vi "Striptest.vi"(1 "Simulation?":bool) -> ()   [LabVIEW 2013]
uses:
  InstrControl/Switching/Switching.lvclass
  InstrControl/SupplyControl/SupplyControl.lvclass
  InstrControl/ProbeStationControl/ProbeStationControl.lvclass
  InstrControl/LCRControl/LCRControl.lvclass
  general_VIs/globals/QC_MeasurementSetup.vi
  striptest/ProbePlan/ProbePlanParams.vi
  general_VIs/globals/QC_RunInformation.vi
  InstrControl/InstrumentSetup.vi
  <vilib>/regexp/Match Regular Expression.xnode
  InstrControl/InstrControl.lvclass
  InstrControl/ArduinoControl/ArduinoControl.lvclass
  <vilib>/Analysis/NI_AALBase.lvlib
panel:
  out "Tab Control":enum32{"Striptest Setup", "Striptest"}(tab)
  in  "Bias Voltage [V]":dbl=-150.0 format="%.1f"
  in  "Frequency [Hz] Setup":i32=1000 caption="Frequency [Hz]" format="%#.3p"
  in  "Minimum fraction\nof good strips":dbl=98.0 format="%.1g"
  in  "Quit":bool
  in  "Continue":bool
  in  "Measurement Configurations":bool
  in  "Pinholes Y/N":bool=TRUE
  in  "Capacitance Y/N":bool=TRUE
  in  "Resistance Y/N":bool=TRUE
  in  "Striptest SMU":string(combo)="Keithley 2410"
  in  "LCR Meter":string(combo)="WayneKerr 6440B"
  in  "Temperature":enum16{"Read Arduino", "Enter manually"}(ring)
  in  "Bias Supply":string(combo)="Keithley 2410"
  in  "Hardware Configurations":bool
  in  "DB Serial No. IN:":string caption="DB Serial No.:"
  in  "User:":string(combo)="Christoph"
  in  "Batch No. IN:":string caption="Batch No.:"
  in  "Device Category IN:":string(combo)="Short Strip" caption="Device Category:"
  in  "Wafer No. IN:":string caption="Wafer No.:"
  in  "From4":u16(ring)
  in  "From3":u16(ring)
  in  "From2":u16(ring)
  in  "From 1":u16(ring) caption="From"
  in  "To4":u16(ring)
  in  "To3":u16(ring)
  in  "To2":u16(ring)
  in  "To 1":u16(ring) caption="To"
  out "Region 1":string caption="Region"
  out "Region2":string
  out "Region3":string
  out "Region4":string
  in  "Enable1":bool
  in  "Enable4":bool
  in  "Enable2":bool
  in  "Enable3":bool
  in  "Pinhole Parameters IN":T1={"Base Voltage"=10.0, "Base Ramp [V/step]"=10.0, "Base Step [ms]"=1000, "High Voltage"=100.0, "High Ramp [V/step]"=100.0, "High Step [ms]"=1000} caption="Pinhole Measurement Parameters"
  in  "Manufacturer:":string(combo)="Hamamatsu"
  in  "Auto ReCheck":bool
  in  "Thresholds:":T2={"Current [nA]"=200.0, "Ccoupl Lo [pF/cm]"=20.0, "Ccoupl Hi [pF/cm]"=33.0, "Rbias Lo [MW]"=1.0, "Rbias Hi [MW]"=2.0}
  in  "Rolling\nCurrent Readout":bool=TRUE
  in  "settling\ndelay [ms]":i32=50
  in  "Pinhole Parameters":T1={"Base Voltage"=10.0, "Base Ramp [V/step]"=10.0, "Base Step [ms]"=1000, "High Voltage"=100.0, "High Ramp [V/step]"=100.0, "High Step [ms]"=1000}
  out "Bias On/Off:":bool
  in  "Auto quit &\nswitch off bias":bool
  out "Sensor No.:":string
  out "Device Category:":string
  out "DB Serial No.:":string
  out "Initiated:":string
  in  "ReCheck":bool
  in  "Save Data":bool
  in  "Abort":bool
  in  "Quit w/o saving":bool
  out "Probing Region:":string
  out "Probe Point:":string
  out "Current [nA]:":dbl
  out "Capacitance [pF]:":dbl
  out "Reistance [MW]:":dbl
  out "Last Probe at:":string
  out "Run Duration:":string
  out "Estimated Completion:":string
  out "Status:":string
  out "Probe Card Channels":i32=32
  in  "Show:":u16(ring)
  out "Defects":i32[][](graph)
  out "% OK:":dbl
  out "# total defects:":i32
  out "# probed":i32
  out "Bad Strip List":i32[](array[numeric])
  out "defect type array":i32[](array[numeric])
  out "Resistance [MW]":cluster{u32, i32, "Array OUT":dbl[]}(graph)
  out "Capacitance [pF]":cluster{u32, i32, "Array OUT":dbl[]}(graph)
  out "Current [nA]":cluster{u32, i32, "Array OUT":dbl[]}(graph)
  out "Current Reference 100V":dbl[](array[numeric])
  out "Current Reference 10V":dbl[](array[numeric])
  out "Single Needle":bool
  out "Z profile":i32[][](array[numeric])
  out "Start Temperature [°C]":dbl
  out "Last Temperature [°C]":dbl
  out "disabled channels":i32[](array[numeric])
  out "Module failed/passed":bool
  out "min scale array":i32[](array[numeric])
  out "max scale array":i32[](array[numeric])
  out "total strip number":u32
  out "Region Indices":i32[](array[numeric])
  out "Current Bias Voltage [V]":dbl
  out "Temperature Progression":T3
  out "probe points per region":i32[](array[numeric])
  # "University of \nCambridge"
  # "Sensor QC: Striptest"
  # "Current [nA]"
  # "Statistical information:"
  # "Pinholes:"
  # "Capacitance [pF]"
  # "Punchthroughs:"
  # "Shorts:"
  # "Opens:"
  # "Rpoly:"
  # "Resistance [MW]"
  # "Implant:"
  # "Current segment:"
  # "Ok  Pinhole at base  Pinhole after ramp  Short  Open  Rbias"
  # "Probe Range"
  # "Measurement Configuration"
  # "Hardware"
  # "DUT Description"
  # "Tests Included"
  # "Current status:"
  # "Measurement parameters:"
  # "DUT & Test Description:"
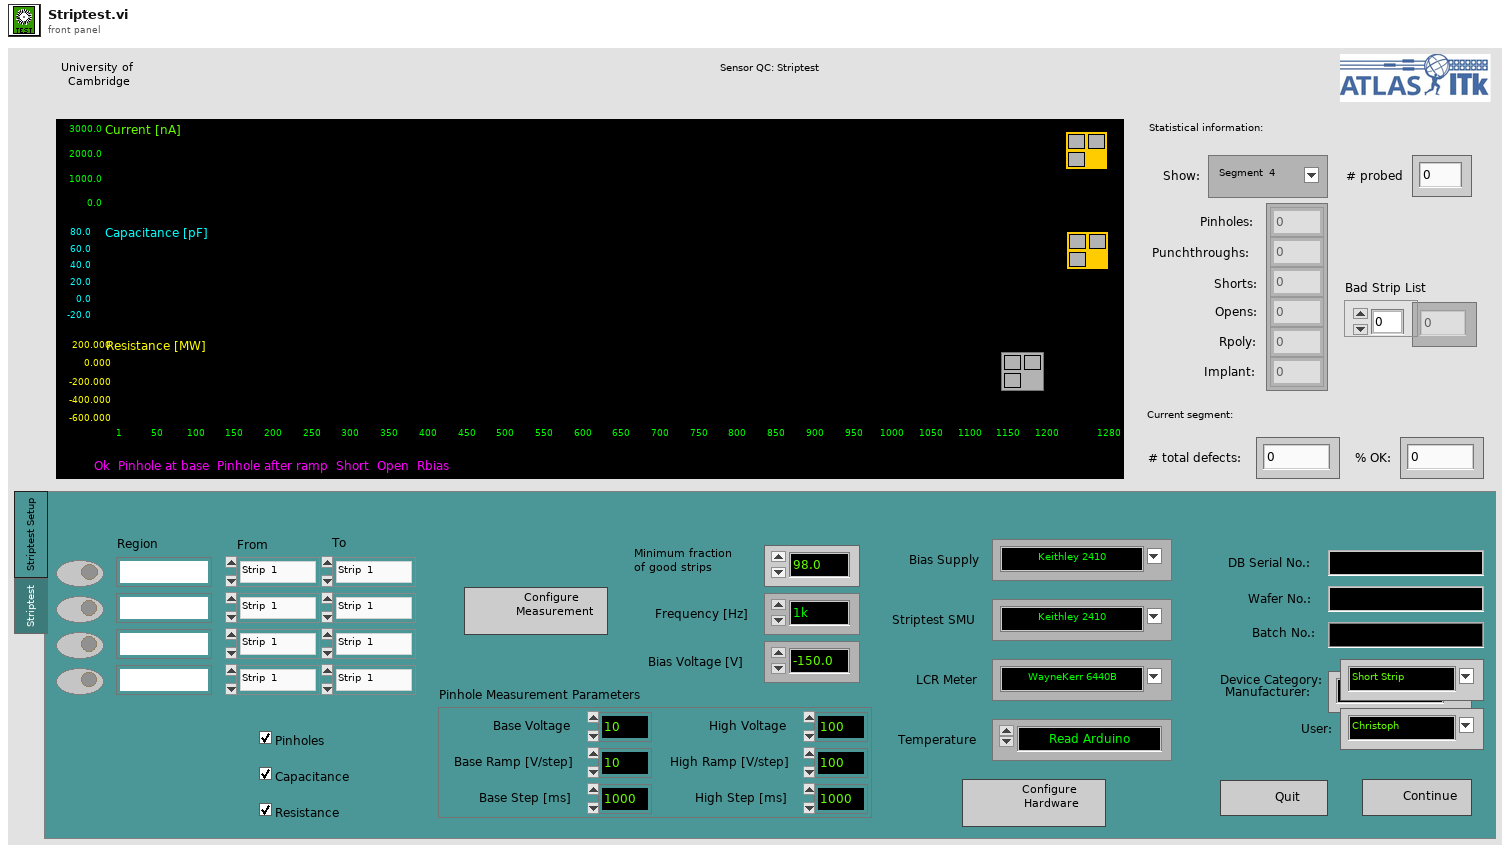
[diagram p1: front panel]
types:
  T1 = cluster{"Base Voltage":dbl, "Base Ramp [V/step]":dbl, "Base Step [ms]":i32, "High Voltage":dbl, "High Ramp [V/step]":dbl, "High Step [ms]":i32}
  T2 = cluster{"Current [nA]":dbl, "Ccoupl Lo [pF/cm]":dbl, "Ccoupl Hi [pF/cm]":dbl, "Rbias Lo [MW]":dbl, "Rbias Hi [MW]":dbl}
  T3 = cluster{"Time Array":string[], "Temperature Array [°C]":dbl[], "Humidity Array [RH %]":dbl[]}
  T4 = enum16{"Supply", "LCR", "Multimeter", "Switching"}
  T5 = enum16{"Reset", "Read Array", "Read Element", "Write Element", "Write Array", "Add Element", "Add Array"}
  T6 = enum16{"Reset", "Ground", "Striptest SMU", "Striptest LCR", "IV", "CV", "Interstrip Cap", "Interstrip Res"}
  T7 = enum16{"Reference measurement", "Baseline correcetion 10V", "Baseline correcetion 100V", "Nothing"}
  T8 = cluster{"Bias Supply":refnum<class "SupplyControl.lvclass">, "SMU":refnum<class "SupplyControl.lvclass">, "LCR":refnum<class "LCRControl.lvclass">, "ProbeStation":refnum<class "ProbeStationControl.lvclass">, "Arduino":refnum<class "ArduinoControl.lvclass">, "Measurement switch":refnum<class "Switching.lvclass">, "Probe Card Channels":i32, "Bias Voltage [V]":dbl, "First strip":i32, "Last strip":i32, "Base Voltage [V]":dbl, "Base Ramp Step [V]":dbl, "Base Ramp Interval [ms]":u32, "High Voltage [V]":dbl, "High Ramp Step [V]":dbl, "High Ramp Interval [ms]":u32, "AC frequency [Hz]":i32, "AC amplitude [V]":dbl, "RC Configuration":u16, "Single Needle":bool, "Temperature Readout":enum16{"Read Arduino", "Enter manually"}, "Fraction of good strips [%]":dbl, "Measurement switch used?":bool, "Matrix X Channels":cluster{"Mux1 C1":i32, "Mux1 C2":i32, "Mux2 C1":i32, "Mux2 C2":i32}, "Pinholes Y/N":bool, "Capacitance Y/N":bool, "Resistance Y/N":bool, "Bias Supply Name":string, "SMU Name":string, "LCR Name":string}
  T9 = cluster{"Institute":string, "Manufacturers":string[], "Devices":string[], "Serialnumbers Lookup DB":string, "Data directory":string, "Backup & screenshot directory":string, "List of known users":string[], "Measurement switch not used":bool, "Measurement Switch":string, "DUT Switch":string, "Rseries IV [MOhm]":string, "Rshunt IV [MOhm]":string, "Rseries CV [MOhm]":string, "DC blocking Cap [µF]":string, "Rseries LCR [MOhm]":string, "Rseries stability [MOhm]":string, "Rshunt stability [MOhm]":string, "Rseries striptest bias [MOhm]":string, "Rseries strip pinhole [MOhm]":string}
  T10 = cluster{"Sensor Serial No.:":string, "Wafer:":string, "Batch:":string, "Manufacturer:":string, "Device Category:":string, "Database Serial No.:":string, "Date Initiated:":string, "Time Initiated:":string, "Test":string, "Probeplan used:":string, "End of Run comment:":string, "User:":string, "Vbias SMU":string, "LCR":string, "Test SMU":string, "Test DMM":string}
  T11 = cluster{"Strip Number OUT":i32, "X0":i32, "Y0":i32, "X1":i32, "Y1":i32, "Xref":dbl, "Yref":dbl, "ProbePlan type":u32, "Inner pads offset":ext, "Outer pads offset":ext, "l_inner":ext, "l_outer":ext, "strip numbering":u16, "Device Orientation":ext, "Stagger offset":i32, "Yoffset":dbl, "Strip pitch":dbl, "Fiducail separation":dbl, "Radius":ext, "Relative strip angles":dbl, "Probeplan description":string, "ProbePlan array":cluster{"Region":string, "ProbePoints":cluster{"X":dbl, "Y":dbl, "Label":string, "CardViable?":bool}[]}[], "Test ProbePoints":cluster{"Regions Enabled":bool[], "From index":u32[], "To index":u32[]}}
  T12 = cluster{"Region":string, "ProbePoints":cluster{"X":dbl, "Y":dbl, "Label":string, "CardViable?":bool}[]}[]
  T13 = cluster{"VISA address":refnum<visa-resource-name>, "T sensor":enum16{"SHT", "DS"}, "Arduino":refnum<class "ArduinoControl.lvclass">}
  T14 = cluster{"X":dbl, "Y":dbl, "Label":string, "CardViable?":bool}[]
  T15 = cluster{"X":dbl, "Y":dbl, "Label":string, "CardViable?":bool}
  T16 = cluster{"pass Rate in %":dbl, "Bad channel list":i32[], "No of bad strips":i32, "Defect description list":i32[], "Number of defects per category":i32[], "Defect lists":string[], "No of channels":i32, "Defect Flag array OUT":i32[][]}
  T17 = cluster{"Hi Cap":dbl, "Lo Cap":dbl, "Current threshold":dbl, "Lo R":dbl, "Hi R":dbl}
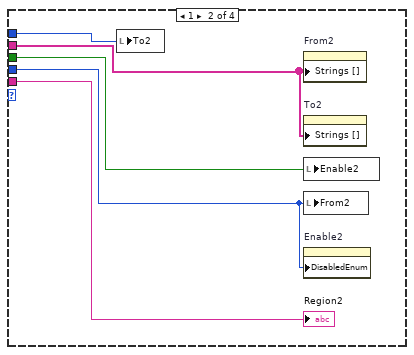
[diagram p3: hidden frame]
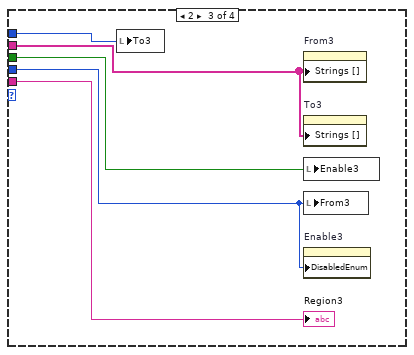
[diagram p4: hidden frame]
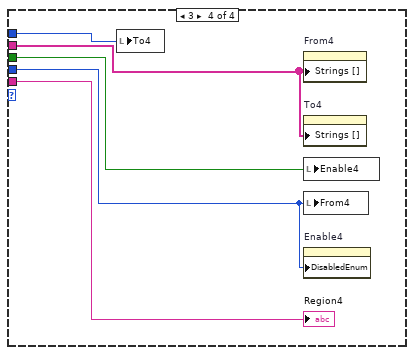
[diagram p5: hidden frame]
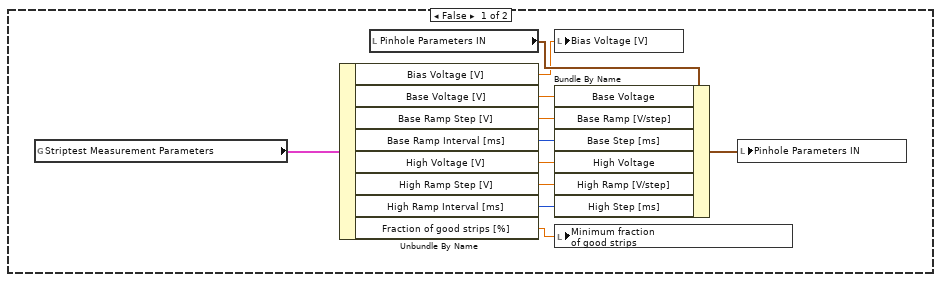
[diagram p7: hidden frame]
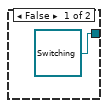
[diagram p9: hidden frame]
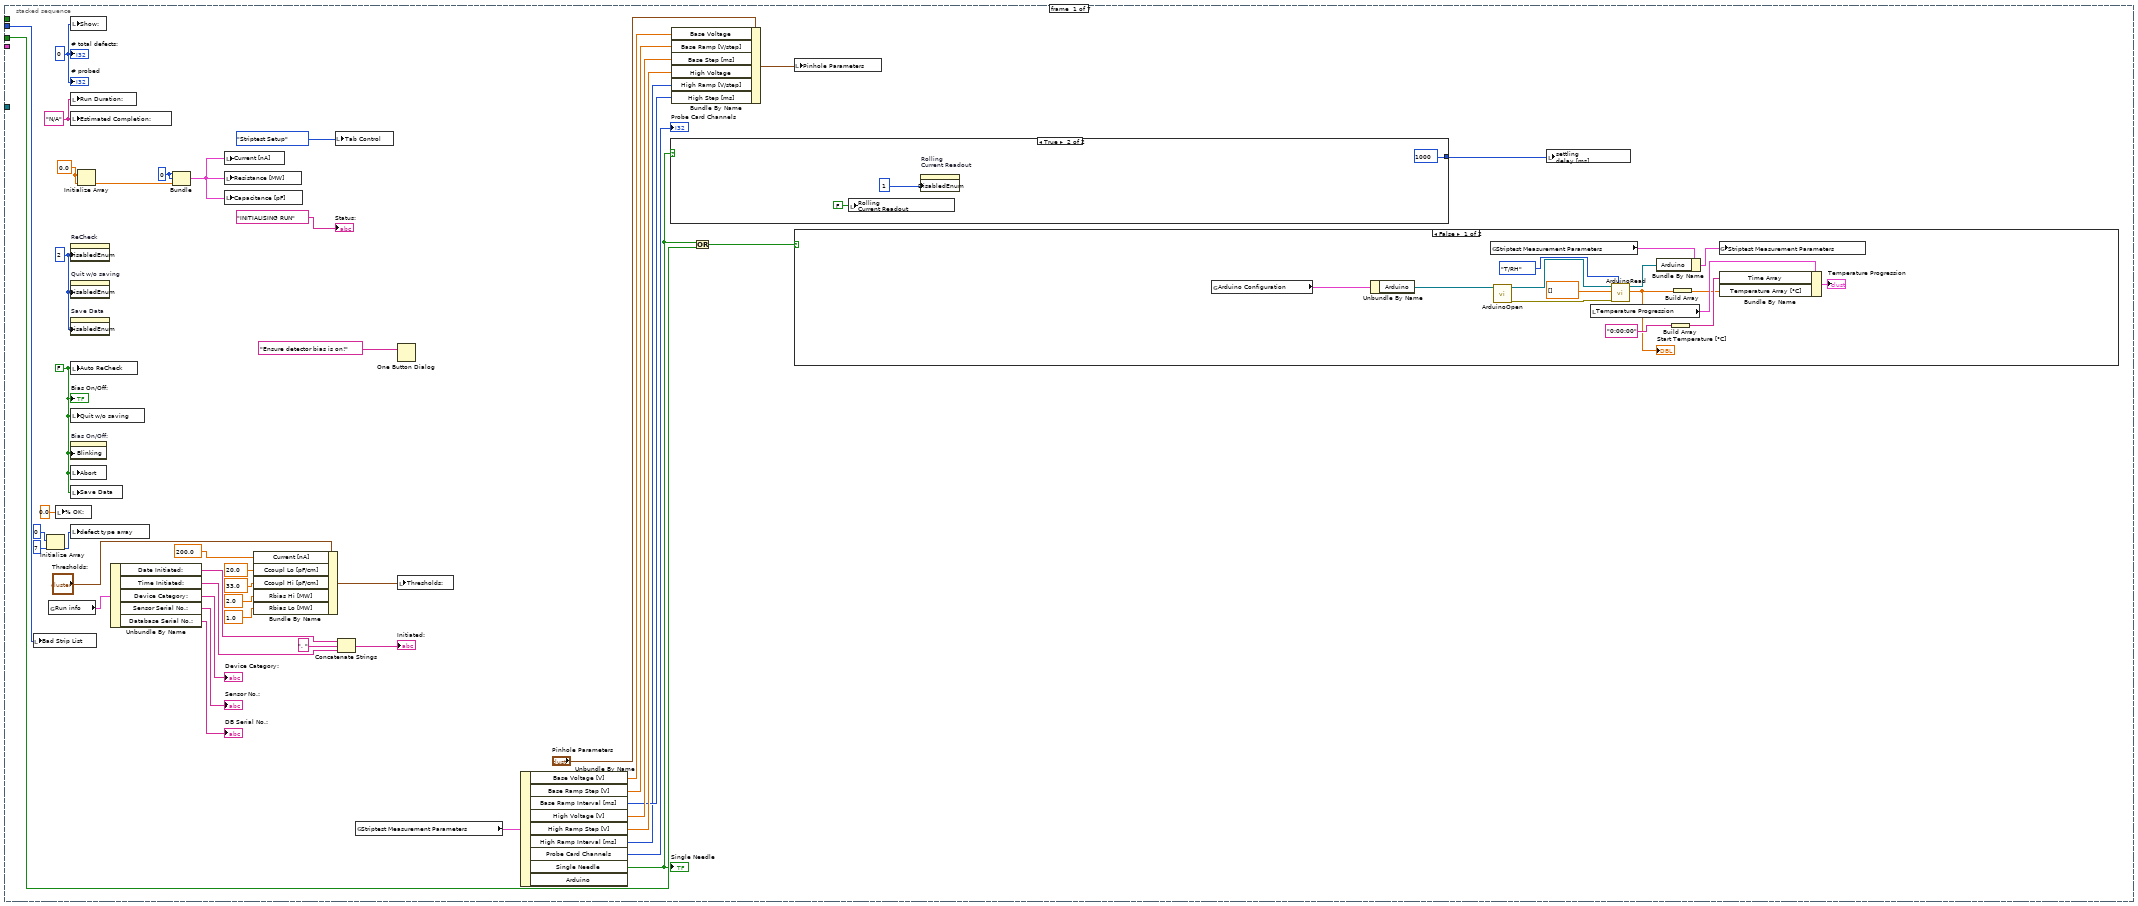
[diagram p10: hidden frame]
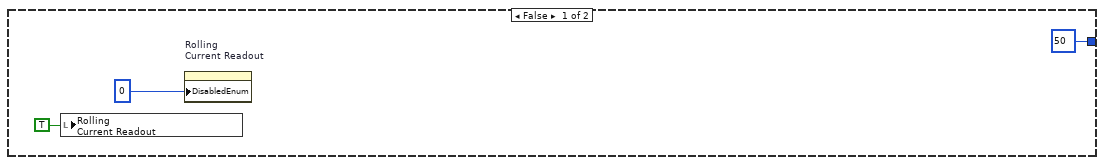
[diagram p11: hidden frame]
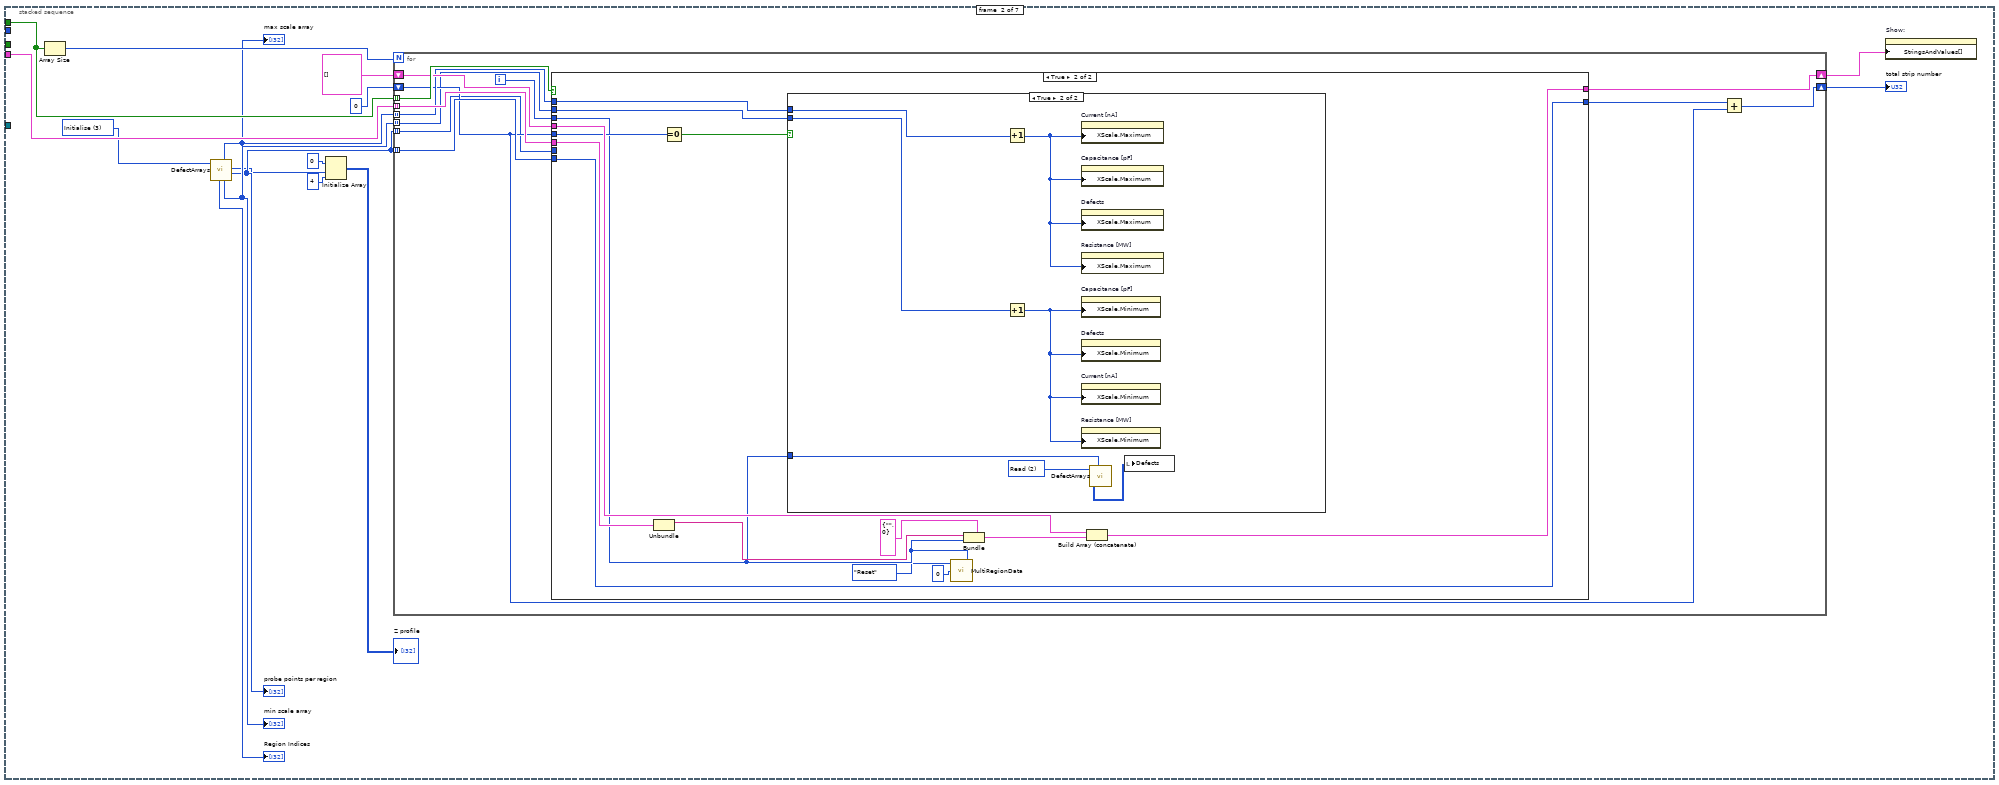
[diagram p13: hidden frame]
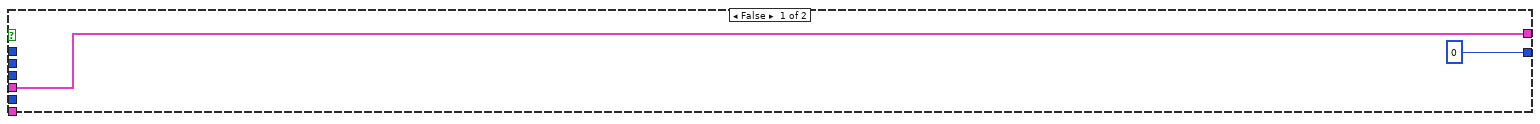
[diagram p14: hidden frame]
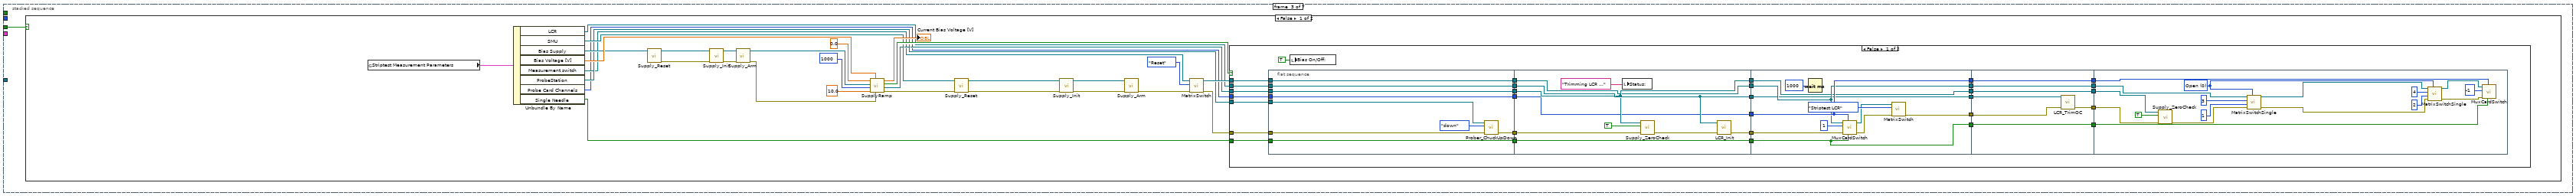
[diagram p16: hidden frame]
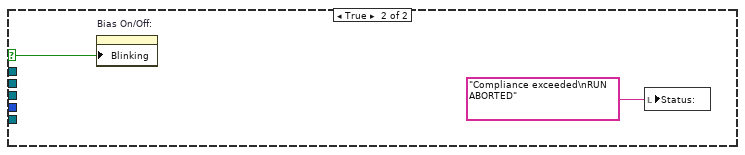
[diagram p17: hidden frame]
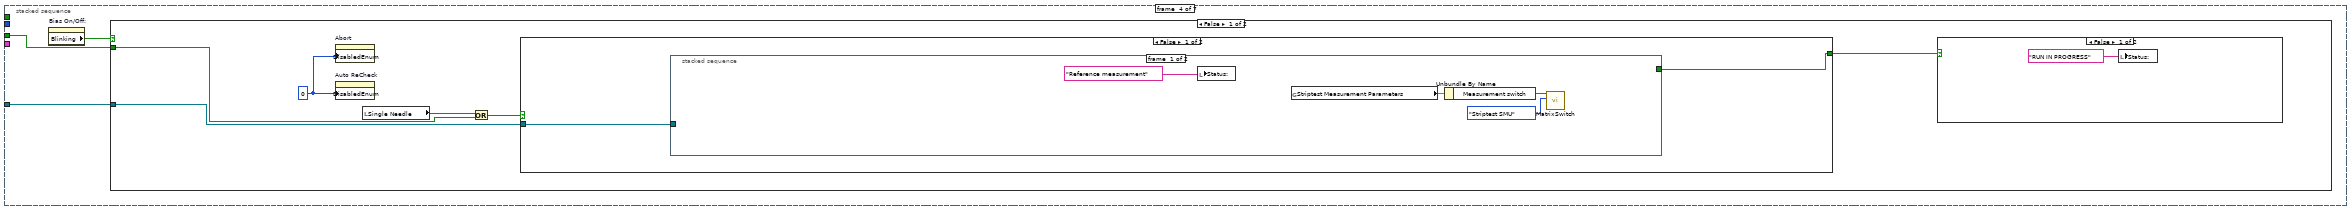
[diagram p19: hidden frame]
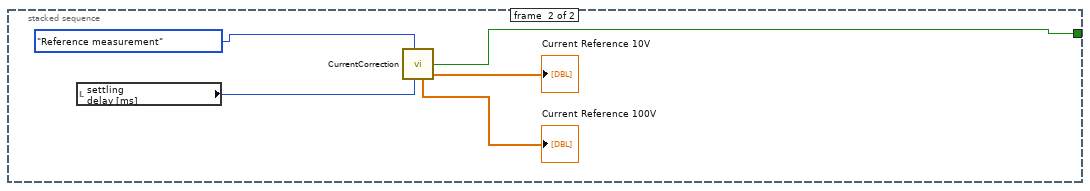
[diagram p20: hidden frame]
diagram:
  n1 = stacked-sequence {
    frame #0 {
      # "Striptest setup"
      n2 = flat-sequence {
        frame #0 {
          w5 = ""
          w6 = 2
          w7 = FALSE
          n3 = property on="Enable4" class="Bool (strict)"("DisabledEnum"=w6) -> ()  [unwired: 2 in, 2 out]
          n4 = property on="Enable1" class="Bool (strict)"("DisabledEnum"=w6) -> ()  [unwired: 2 in, 2 out]
          n5 = property on="Enable2" class="Bool (strict)"("DisabledEnum"=w6) -> ()  [unwired: 2 in, 2 out]
          n6 = property on="Enable3" class="Bool (strict)"("DisabledEnum"=w6) -> ()  [unwired: 2 in, 2 out]
          n7 = local write "Region 1"(w5) -> ()
          n8 = local write "Region2"(w5) -> ()
          n9 = local write "Region3"(w5) -> ()
          n10 = local write "Region4"(w5) -> ()
          n11 = local write "Enable2"(w7) -> ()
          n12 = local write "Enable1"(w7) -> ()
          n13 = local write "Enable3"(w7) -> ()
          n14 = local write "Enable4"(w7) -> ()
          n15 = call <vilib>:"Open Sessions.vi"() -> ("Array of Refnums"=w2:refnum<visa-resource-name>[])  [unwired: 2 in]
          n16 = for {
            tunnel: w2 -> [w13] mode=indexing
            tunnel: [w12] -> w1
            n17 = VISA Close(VISA resource name=w13) -> (error out=w12:errorcluster)  [unwired: 1 in]
          }
          n18 = call "SelectStriptestProber.vi"("error in (no error)"=w1) -> ("error out"=w8:errorcluster, "ProbeStationControl out"=w9:refnum<class "ProbeStationControl.lvclass">)  [unwired: 9 in]
          n19 = global read "QC_MeasurementSetup.vi" "Striptest Measurement Parameters"() -> (w11:T8)
          n20 = call "InitialiseProbeplan.vi"("error in (no error)"=w8, "ProbeStationControl in"=w9) -> ()  [unwired: 8 in, 2 out]
          n21 = Bundle By Name(cluster=w11, "ProbeStation"=w9) -> (w10:T8)
          n22 = global write "QC_MeasurementSetup.vi" "Striptest Measurement Parameters"(w10) -> ()
          n23 = call "GetLocalConfiguration.vi"() -> ()  [unwired: 3 in, 1 out]
          n24 = call "GetGlobalDefaultConfiguration.vi"("Read defaults?"=TRUE) -> ()  [unwired: 3 in]
          "Tab Control" <- enum32{"Striptest Setup", "Striptest"}."Striptest Setup" ("Tab Control")
        }
        frame #1 {
          n25 = flat-sequence {
            frame #0 {
              n26 = call "SerialNo.vi"("DB serial number IN"="", "Run uninterrupted?"=FALSE) -> ()  [unwired: 6 in, 2 out]
              n27 = global read "QC_RunInformation.vi" "LocalConfiguration"() -> (w49:T9)
              n28 = Unbundle By Name(w49) -> ("List of known users"=w51:string[], "Devices"=w46:string[], "Manufacturers"=w45:string[])
              n29 = property on="Device Category IN:" class="CmbBox"("Strings[]"=w46) -> ()  [unwired: 2 in, 2 out]
              n30 = property on="Manufacturer:" class="CmbBox"("Strings[]"=w45) -> ()  [unwired: 2 in, 2 out]
              n31 = Index Array(array=w46, index=0) -> (element=w43:string)
              n32 = Index Array(array=w45, index=0) -> (element=w44:string)
              n33 = property on="User:" class="CmbBox"("Strings[]"=w51, "AllowUndefStrs"=TRUE) -> ()  [unwired: 2 in, 2 out]
              n34 = local write "Device Category IN:"(w43) -> ()
              n35 = local write "Manufacturer:"(w44) -> ()
            }
            frame #1 {
              n36 = global read "QC_RunInformation.vi" "Run info"() -> (w54:T10)
              n37 = Unbundle By Name(w54) -> ("Wafer:"=w55:string, "Batch:"=w56:string, "Manufacturer:"=w57:string, "Device Category:"=w58:string, "Database Serial No.:"=w59:string)
              n38 = local write "Manufacturer:"(w57) -> ()
              n39 = local write "Device Category IN:"(w58) -> ()
              n40 = local write "DB Serial No. IN:"(w59) -> ()
              n41 = local write "Wafer No. IN:"(w55) -> ()
              n42 = local write "Batch No. IN:"(w56) -> ()
            }
          }
          n43 = global read "QC_RunInformation.vi" "Run info"() -> (w33:T10)
          n44 = call "InstrumentNames.vi"("Instrument type"=T4."Supply") -> ("error out"=w36:errorcluster, "Instrument names"=w38:string[])  [unwired: 9 in]
          n45 = global read "ProbePlanParams.vi" "ProbePlan Parameters IN"() -> (w42:T11)
          n46 = property on="Bias Supply" class="CmbBox"("Strings[]"=w38) -> ()  [unwired: 2 in, 2 out]
          n47 = property on="Striptest SMU" class="CmbBox"("Strings[]"=w38) -> ()  [unwired: 2 in, 2 out]
          n48 = Bundle By Name(cluster=w33, "Test"="STRIPTEST") -> (w34:T10)
          n49 = global write "QC_RunInformation.vi" "Run info"(w34) -> ()
          n50 = call "InstrumentNames.vi"("error in (no error)"=w36, "Instrument type"=T4."LCR") -> ("Instrument names"=w35:string[])  [unwired: 8 in, 1 out]
          n51 = property on="LCR Meter" class="CmbBox"("Strings[]"=w35) -> ()  [unwired: 2 in, 2 out]
          n52 = global read "QC_MeasurementSetup.vi" "Striptest Measurement Parameters"() -> (w32:T8)
          n53 = Unbundle By Name(w42) -> ("ProbePlan array"=w41:T12)
          n54 = Array Size(array=w41) -> (size(s)=w40:i32)
          n55 = for {
            N: w40 -> [_]
            tunnel: w41 -> [w61]
            tunnel: w41 -> [w65] mode=indexing
            i -> [w68]
            n56 = Unbundle(w65) -> ("Region"=w64:string)  [unwired: 1 out]
            n57 = call "GetLabels.vi"("Array"=w61) -> ("Strip Labels"=w60:string[])  [unwired: 3 out]
            n58 = Array Size(array=w60) -> (size(s)=w63:i32)
            n59 = Decrement(x=w63) -> (x-1=w62:i32)
            n60 = case shown="0, Default" w68 {
              tunnel: TRUE -> [w73 w77 w83 w88]
              tunnel: 0 -> [w69 w75 w79 w85]
              tunnel: w64 -> [w71 w76 w81 w86]
              tunnel: w60 -> [w70 w74 w80 w84]
              tunnel: w62 -> [w72 w78 w82 w87]
              frame 0, Default {
                n61 = local write "To 1"(w72) -> ()
                n62 = property on="To 1" class="Ring (strict)"("Strings []"=w70) -> ()  [unwired: 2 in, 2 out]
                n63 = property on="From 1" class="Ring (strict)"("Strings []"=w70) -> ()  [unwired: 2 in, 2 out]
                n64 = local write "Enable1"(w73) -> ()
                n65 = local write "From 1"(w69) -> ()
                n66 = property on="Enable1" class="Bool (strict)"("DisabledEnum"=w69) -> ()  [unwired: 2 in, 2 out]
                "Region 1" <- w71
              }
              frame 1 {
                n67 = local write "To2"(w78) -> ()
                n68 = property on="From2" class="Ring (strict)"("Strings []"=w74) -> ()  [unwired: 2 in, 2 out]
                n69 = property on="To2" class="Ring (strict)"("Strings []"=w74) -> ()  [unwired: 2 in, 2 out]
                n70 = local write "Enable2"(w77) -> ()
                n71 = local write "From2"(w75) -> ()
                n72 = property on="Enable2" class="Bool (strict)"("DisabledEnum"=w75) -> ()  [unwired: 2 in, 2 out]
                "Region2" <- w76
              }
              frame 2 {
                n73 = local write "To3"(w82) -> ()
                n74 = property on="From3" class="Ring (strict)"("Strings []"=w80) -> ()  [unwired: 2 in, 2 out]
                n75 = property on="To3" class="Ring (strict)"("Strings []"=w80) -> ()  [unwired: 2 in, 2 out]
                n76 = local write "Enable3"(w83) -> ()
                n77 = local write "From3"(w79) -> ()
                n78 = property on="Enable3" class="Bool (strict)"("DisabledEnum"=w79) -> ()  [unwired: 2 in, 2 out]
                "Region3" <- w81
              }
              frame 3 {
                n79 = local write "To4"(w87) -> ()
                n80 = property on="From4" class="Ring (strict)"("Strings []"=w84) -> ()  [unwired: 2 in, 2 out]
                n81 = property on="To4" class="Ring (strict)"("Strings []"=w84) -> ()  [unwired: 2 in, 2 out]
                n82 = local write "Enable4"(w88) -> ()
                n83 = local write "From4"(w85) -> ()
                n84 = property on="Enable4" class="Bool (strict)"("DisabledEnum"=w85) -> ()  [unwired: 2 in, 2 out]
                "Region4" <- w86
              }
            }
          }
          n85 = Unbundle By Name(w32) -> ("Probe Card Channels"=w31:i32, "Bias Voltage [V]"=w22:dbl, "Base Voltage [V]"=w28:dbl, "Base Ramp Step [V]"=w27:dbl, "Base Ramp Interval [ms]"=w26:u32, "High Voltage [V]"=w25:dbl, "High Ramp Step [V]"=w24:dbl, "High Ramp Interval [ms]"=w23:u32, "Single Needle"=w21:bool, "Temperature Readout"=w20:enum16{"Read Arduino", "Enter manually"}, "Fraction of good strips [%]"=w19:dbl, "AC frequency [Hz]"=w18:i32, "Pinholes Y/N"=w17:bool, "Capacitance Y/N"=w16:bool, "Resistance Y/N"=w15:bool)
          n86 = local read "Pinhole Parameters IN"() -> (w30:T1)
          n87 = Bundle By Name(cluster=w30, "Base Voltage"=w28, "Base Ramp [V/step]"=w27, "Base Step [ms]"=w26, "High Voltage"=w25, "High Ramp [V/step]"=w24, "High Step [ms]"=w23) -> (w29:T1)
          n88 = local write "Probe Card Channels"(w31) -> ()
          n89 = local write "Bias Voltage [V]"(w22) -> ()
          n90 = local write "Single Needle"(w21) -> ()
          n91 = local write "Temperature"(w20) -> ()
          n92 = local write "Minimum fraction\nof good strips"(w19) -> ()
          n93 = local write "Frequency [Hz] Setup"(w18) -> ()
          n94 = local write "Pinholes Y/N"(w17) -> ()
          n95 = local write "Capacitance Y/N"(w16) -> ()
          n96 = local write "Resistance Y/N"(w15) -> ()
          n97 = local write "Pinhole Parameters IN"(w29) -> ()
        }
        frame #2 {
          n98 = while {
            shift-right: [w92] -> _
            shift-left: FALSE -> [w94]
            stop <- "Continue" stop-if-true
            n99 = Stop(stop? (T)="Quit") -> ()
            n100 = local read "DB Serial No. IN:"() -> (w98:string)
            n101 = local read "Wafer No. IN:"() -> (w100:string)
            n102 = local read "Batch No. IN:"() -> (w99:string)
            n103 = Empty String/Path?(string/path=w100) -> (empty?=w97:bool)
            n104 = Empty String/Path?(string/path=w99) -> (empty?=w96:bool)
            n105 = Empty String/Path?(string/path=w98) -> (empty?=w95:bool)
            n106 = case shown="True" "Measurement Configurations" {
              frame False {
              }
              frame True {
                n107 = Two Button Dialog(message="With this, you will change QC measurement parameters defined by the collaboration!\n\nDo you really wish to continue?", 2:"YES") -> (T button?=w106:bool)  [unwired: 1 in]
                n108 = case shown="True" w106 {
                  frame False {
                    n109 = global read "QC_MeasurementSetup.vi" "Striptest Measurement Parameters"() -> (w119:T8)
                    n110 = Unbundle By Name(w119) -> ("Bias Voltage [V]"=w109:dbl, "Base Voltage [V]"=w116:dbl, "Base Ramp Step [V]"=w115:dbl, "Base Ramp Interval [ms]"=w114:u32, "High Voltage [V]"=w113:dbl, "High Ramp Step [V]"=w112:dbl, "High Ramp Interval [ms]"=w111:u32, "Fraction of good strips [%]"=w110:dbl)
                    n111 = local read "Pinhole Parameters IN"() -> (w118:T1)
                    n112 = local write "Bias Voltage [V]"(w109) -> ()
                    n113 = Bundle By Name(cluster=w118, "Base Voltage"=w116, "Base Ramp [V/step]"=w115, "Base Step [ms]"=w114, "High Voltage"=w113, "High Ramp [V/step]"=w112, "High Step [ms]"=w111) -> (w117:T1)
                    n114 = local write "Minimum fraction\nof good strips"(w110) -> ()
                    n115 = local write "Pinhole Parameters IN"(w117) -> ()
                  }
                  frame True {
                    n116 = global read "QC_MeasurementSetup.vi" "Striptest Measurement Parameters"() -> (w130:T8)
                    n117 = Unbundle By Name("Pinhole Parameters IN") -> ("Base Voltage"=w126:dbl, "Base Ramp [V/step]"=w125:dbl, "Base Step [ms]"=w124:i32, "High Voltage"=w123:dbl, "High Ramp [V/step]"=w122:dbl, "High Step [ms]"=w121:i32)
                    n118 = Bundle By Name(cluster=w130, "Bias Voltage [V]"="Bias Voltage [V]", "Base Voltage [V]"=w126, "Base Ramp Step [V]"=w125, "Base Ramp Interval [ms]"=w124, "High Voltage [V]"=w123, "High Ramp Step [V]"=w122, "High Ramp Interval [ms]"=w121, "Fraction of good strips [%]"="Minimum fraction\nof good strips") -> (w129:T8)
                    n119 = global write "QC_MeasurementSetup.vi" "Striptest Measurement Parameters"(w129) -> ()
                  }
                }
              }
            }
            n120 = case shown="True" "Hardware Configurations" {
              tunnel: [w131 w132] -> w92
              tunnel: w94 -> [w131 _]
              frame False {
              }
              frame True {
                n121 = call "HardwareConfiguration.vi"() -> ("configured?"=w132:bool)  [unwired: 11 in]
              }
            }
            n122 = Compound Arithmetic op=OR(w97, w96, w95) -> (invert w101:bool)
            n123 = Select(t=0, s=w101, f=2) -> (s? t:f=w91:i32)
            n124 = property on="Continue" class="Bool"("DisabledEnum"=w91) -> ()  [unwired: 2 in, 2 out]
          }
        }
        frame #3 {
          w136 = TRUE
          w164 = T4."Supply" ("Instrument type")
          n125 = global read "QC_RunInformation.vi" "LocalConfiguration"() -> (w139:T9)
          n126 = call "InstrumentSelection.vi"("Verify GPIB address"=w136, "Instrument type"=w164, "Instrument name IN"="Bias Supply") -> ("error out"=w170:errorcluster, "Instrument name OUT"=w141:string, "Supply"=w165:refnum<class "SupplyControl.lvclass">)  [unwired: 3 in, 3 out]
          n127 = call "InstrumentSelection.vi"("error in (no error)"=w170, "Verify GPIB address"=w136, "Instrument type"=w164, "Instrument name IN"="Striptest SMU") -> ("error out"=w160:errorcluster, "Instrument name OUT"=w140:string, "Supply"=w162:refnum<class "SupplyControl.lvclass">)  [unwired: 2 in, 3 out]
          n128 = Unbundle By Name(w139) -> ("Measurement Switch"=w138:string, "Measurement switch not used"=w137:bool)
          n129 = global read "ProbePlanParams.vi" "ProbePlan Parameters IN"() -> (w191:T11)
          n130 = Build Array("Enable1", "Enable2", "Enable3", "Enable4") -> (w189:bool[])
          n131 = Build Array("From 1", "From2", "From3", "From4") -> (w188:u16[])
          n132 = Build Array("To 1", "To2", "To3", "To4") -> (w187:u16[])
          n133 = Bundle By Name(cluster=w191, "Test ProbePoints.Regions Enabled"=w189, "Test ProbePoints.From index"=w188, "Test ProbePoints.To index"=w187) -> (w190:T11)
          n134 = Unbundle By Name(w191) -> ("Probeplan description"=w153:string)
          n135 = Concatenate Strings("Batch No. IN:", "-", "Wafer No. IN:") -> (w145:string)
          n136 = call "InstrumentSelection.vi"("error in (no error)"=w160, "Verify GPIB address"=w136, "Instrument type"=T4."LCR", "Instrument name IN"="LCR Meter") -> ("error out"=w135:errorcluster, "Instrument name OUT"=w142:string, "LCR"=w161:refnum<class "LCRControl.lvclass">)  [unwired: 2 in, 3 out]
          n137 = Not(x=w137) -> (.not. x?=w133:bool)
          n138 = global read "QC_RunInformation.vi" "Run info"() -> (w168:T10)
          n139 = Get Date/Time String(date format (0)=enum16{"short", "long", "abbreviated"}."abbreviated", want seconds? (F)=TRUE) -> (date string=w155:string, time string=w154:string)  [unwired: 1 in]
          n140 = global write "ProbePlanParams.vi" "ProbePlan Parameters IN"(w190) -> ()
          n141 = case shown="True" w133 {
            tunnel: w135 -> [_ w196]
            tunnel: [refnum<class "Switching.lvclass"> refnum ("Switching") w195] -> w134
            tunnel: w136 -> [_ w194]
            tunnel: w138 -> [_ w193]
            frame False {
            }
            frame True {
              n142 = call "InstrumentSelection.vi"("error in (no error)"=w196, "Verify GPIB address"=w194, "Instrument type"=T4."Switching", "Instrument name IN"=w193) -> ("Switching"=w195:refnum<class "Switching.lvclass">)  [unwired: 2 in, 5 out]
            }
          }
          n143 = Bundle By Name(cluster=w168, "Sensor Serial No.:"=w145, "Wafer:"="Wafer No. IN:", "Batch:"="Batch No. IN:", "Manufacturer:"="Manufacturer:", "Device Category:"="Device Category IN:", "Database Serial No.:"="DB Serial No. IN:", "Date Initiated:"=w155, "Time Initiated:"=w154, "Vbias SMU"=w141, "LCR"=w142, "Test SMU"=w140, "Probeplan used:"=w153, "User:"="User:") -> (w174:T10)
          n144 = global read "QC_MeasurementSetup.vi" "Striptest Measurement Parameters"() -> (w167:T8)
          n145 = global write "QC_RunInformation.vi" "Run info"(w174) -> ()
          n146 = Bundle By Name(cluster=w167, "Bias Supply"=w165, "SMU"=w162, "LCR"=w161, "Measurement switch"=w134, "Measurement switch used?"=w133, "Temperature Readout"="Temperature", "AC frequency [Hz]"="Frequency [Hz] Setup", "Pinholes Y/N"="Pinholes Y/N", "Capacitance Y/N"="Capacitance Y/N", "Resistance Y/N"="Resistance Y/N") -> (w166:T8)
          n147 = global write "QC_MeasurementSetup.vi" "Striptest Measurement Parameters"(w166) -> ()
        }
      }
    }
    frame #1 {
      # "Striptest measurement procedure"
      n148 = global read "QC_MeasurementSetup.vi" "Striptest Measurement Parameters"() -> (w198:T8)
      n149 = global read "ProbePlanParams.vi" "ProbePlan Parameters IN"() -> (w205:T11)
      n150 = Unbundle By Name(w205) -> ("Test ProbePoints.Regions Enabled"=w201:bool[], "ProbePlan array"=w200:T12)
      n151 = Unbundle By Name(w198) -> ("ProbeStation"=w199:refnum<class "ProbeStationControl.lvclass">)
      n152 = Initialize Array(0) -> (w203:i32[])  [unwired: 1 in]
      n153 = stacked-sequence {
        tunnel: w203 -> [w230 _ _ _ w466 _ _]
        tunnel: "Simulation?" -> [w225 _ w323 w444 _ w1073 w1131]
        tunnel: w201 -> [_ w286 _ _ w469 _ w1130]
        tunnel: w200 -> [_ w285 _ _ w467 _ _]
        tunnel: w199 -> [_ _ _ w442 _ w1072 _]
        frame #0 {
          w232 = "N/A"
          w227 = FALSE
          w240 = 2
          w233 = 0
          w249 = 0
          w248 = 0.0
          n154 = local write "Bad Strip List"(w230) -> ()
          n155 = Initialize Array(0, 7 ("Dimension Size")) -> (w228:i32[])
          n156 = global read "QC_RunInformation.vi" "Run info"() -> (w246:T10)
          n157 = local write "% OK:"(0.0) -> ()
          n158 = local write "Show:"(w233) -> ()
          n159 = local write "Run Duration:"(w232) -> ()
          n160 = local write "Estimated Completion:"(w232) -> ()
          n161 = property on="ReCheck" class="Bool"("DisabledEnum"=w240) -> ()  [unwired: 2 in, 2 out]
          n162 = property on="Quit w/o saving" class="Bool (strict)"("DisabledEnum"=w240) -> ()  [unwired: 2 in, 2 out]
          n163 = property on="Save Data" class="Bool (strict)"("DisabledEnum"=w240) -> ()  [unwired: 2 in, 2 out]
          n164 = local write "Auto ReCheck"(w227) -> ()
          n165 = local write "Quit w/o saving"(w227) -> ()
          n166 = property on="Bias On/Off:" class="Bool (strict)"("Blinking"=w227) -> ()  [unwired: 2 in, 2 out]
          n167 = local write "Abort"(w227) -> ()
          n168 = local write "Save Data"(w227) -> ()
          n169 = local write "defect type array"(w228) -> ()
          n170 = Initialize Array(w248, w248) -> (w250:dbl[])
          n171 = Unbundle By Name(w246) -> ("Date Initiated:"=w208:string, "Time Initiated:"=w206:string, "Device Category:"=→"Device Category:":string, "Sensor Serial No.:"=→"Sensor No.:":string, "Database Serial No.:"=→"DB Serial No.:":string)
          n172 = Bundle(w249, w249, w250) -> (w247:cluster{i32, i32, dbl[]})  [unwired: 1 in]
          n173 = local write "Current [nA]"(w247) -> ()
          n174 = local write "Resistance [MW]"(w247) -> ()
          n175 = local write "Capacitance [pF]"(w247) -> ()
          n176 = Bundle By Name(cluster="Thresholds:", "Current [nA]"=200.0 ("CapLo"), "Ccoupl Lo [pF/cm]"=20.0 ("CapLo"), "Ccoupl Hi [pF/cm]"=33.0 ("CapHi"), "Rbias Hi [MW]"=2.0 ("Rpolyhi"), "Rbias Lo [MW]"=1.0 ("RpolyLo")) -> (w238:T2)
          n177 = local write "Tab Control"(enum32{"Striptest Setup", "Striptest"}."Striptest Setup" ("Tab Control")) -> ()
          n178 = Concatenate Strings(w208, ", ", w206) -> (→"Initiated:":string)
          n179 = global read "QC_MeasurementSetup.vi" "Striptest Measurement Parameters"() -> (w213:T8)
          n180 = One Button Dialog(message="Ensure detector bias is on!") -> ()  [unwired: 1 in, 1 out]
          n181 = local write "Thresholds:"(w238) -> ()
          n182 = Unbundle By Name(w213) -> ("Base Voltage [V]"=w221:dbl, "Base Ramp Step [V]"=w222:dbl, "Base Ramp Interval [ms]"=w218:u32, "High Voltage [V]"=w219:dbl, "High Ramp Step [V]"=w220:dbl, "High Ramp Interval [ms]"=w217:u32, "Probe Card Channels"=→"Probe Card Channels":i32, "Single Needle"=w212:bool)  [unwired: 1 out]
          "Single Needle" <- w212
          n183 = case shown="True" w212 {
            tunnel: [50 1000] -> w214
            frame False {
              n184 = local write "Rolling\nCurrent Readout"(TRUE) -> ()
              n185 = property on="Rolling\nCurrent Readout" class="Bool (strict)"("DisabledEnum"=0) -> ()  [unwired: 2 in, 2 out]
            }
            frame True {
              n186 = local write "Rolling\nCurrent Readout"(FALSE) -> ()
              n187 = property on="Rolling\nCurrent Readout" class="Bool (strict)"("DisabledEnum"=1) -> ()  [unwired: 2 in, 2 out]
            }
          }
          n188 = Bundle By Name(cluster="Pinhole Parameters", "Base Voltage"=w221, "Base Ramp [V/step]"=w222, "Base Step [ms]"=w219, "High Voltage"=w220, "High Ramp [V/step]"=w217, "High Step [ms]"=w218) -> (w223:T1)
          n189 = Or(x=w212, y=w225) -> (x .or. y?=w224:bool)
          n190 = local write "Pinhole Parameters"(w223) -> ()
          n191 = case shown="False" w224 {
            frame False {
              n192 = global read "InstrumentSetup.vi" "Arduino Configuration"() -> (w271:T13)
              n193 = Unbundle By Name(w271) -> ("Arduino"=w263:refnum<class "ArduinoControl.lvclass">)
              n194 = global read "QC_MeasurementSetup.vi" "Striptest Measurement Parameters"() -> (w259:T8)
              n195 = call "ArduinoOpen.vi"("ArduinoControl in"=w263) -> ("error out"=w261:errorcluster, "ArduinoControl out"=w262:refnum<class "ArduinoControl.lvclass">)  [unwired: 9 in]
              n196 = local read "Temperature Progression"() -> (w270:T3)
              n197 = call "ArduinoRead.vi"("Arduino function"=enum16{"T/RH", "Interlock", "Edgesense"}."T/RH", "error in (no error)"=w261, "Temperature IN"=dbl[] [], "ArduinoControl in"=w262) -> ("Temperature [°C]"=w265:dbl, "ArduinoControl out"=w257:refnum<class "ArduinoControl.lvclass">)  [unwired: 2 in, 4 out]
              "Start Temperature [°C]" <- w265
              n198 = Bundle By Name(cluster=w259, "Arduino"=w257) -> (w258:T8)
              n199 = Build Array("0:00:00") -> (w266:string[])
              n200 = Build Array(w265) -> (w264:dbl[])
              n201 = global write "QC_MeasurementSetup.vi" "Striptest Measurement Parameters"(w258) -> ()
              n202 = Bundle By Name(cluster=w270, "Time Array"=w266, "Temperature Array [°C]"=w264) -> (→"Temperature Progression":T3)
            }
            frame True {
            }
          }
          n203 = local write "settling\ndelay [ms]"(w214) -> ()
          "# total defects:" <- w233
          "# probed" <- w233
          "Status:" <- "INITIALISING RUN"
          "Bias On/Off:" <- w227
        }
        frame #1 {
          w281 = u16 3 items=["Nothing", "Write", "Read", "Initialise"] ("action")
          n204 = Array Size(array=w286) -> (size(s)=w287:i32)
          n205 = call "DefectArrays.vi"("action"=w281) -> ("Region Indices"=→"Region Indices":i32[], "To"=w280:i32[], "max. No. of points in region"=w272:i32, "From"=w279:i32[], "No. of points in region"=w274:i32[])  [unwired: 2 in, 3 out]
          "max scale array" <- w280
          "min scale array" <- w279
          "probe points per region" <- w274
          n206 = Initialize Array(0, w272, 4) -> (→"Z profile":i32[][])
          n207 = for {
            N: w287 -> [_]
            tunnel: w286 -> [w299] mode=indexing
            shift-right: [w298] -> w284
            shift-left: cluster{string, i32}[] [] -> [w297]
            tunnel: w285 -> [w296] mode=indexing
            tunnel: w274 -> [w291] mode=indexing
            tunnel: w280 -> [w292] mode=indexing
            tunnel: w279 -> [w289] mode=indexing
            shift-right: [w293] -> w283
            shift-left: 0 -> [w290]
            tunnel: w274 -> [w288] mode=indexing
            i -> [w294]
            n208 = case shown="True" w299 {
              tunnel: w297 -> [w300 w314]
              tunnel: [w300 w313] -> w298
              tunnel: w296 -> [_ w315]
              tunnel: [0 w309] -> w295
              tunnel: w294 -> [_ w306]
              tunnel: w292 -> [_ w311]
              tunnel: w289 -> [_ w310]
              tunnel: w291 -> [_ w309]
              tunnel: w290 -> [_ w308]
              tunnel: w288 -> [_ _]
              frame False {
              }
              frame True {
                n209 = Unbundle(w315) -> ("Region"=w307:string)  [unwired: 1 out]
                n210 = Equal To 0?(x=w308) -> (x = 0?=w312:bool)
                n211 = case shown="True" w312 {
                  tunnel: w311 -> [_ w317]
                  tunnel: w310 -> [_ w319]
                  tunnel: w306 -> [_ w320]
                  frame False {
                  }
                  frame True {
                    w322 = u16 2 items=["Nothing", "Write", "Read", "Initialise"] ("action")
                    n212 = Increment(x=w317) -> (x+1=w316:i32)
                    n213 = Increment(x=w319) -> (x+1=w318:i32)
                    n214 = property on="Current [nA]" class="WFGraph (strict)"("XScale.Maximum"=w316) -> ()  [unwired: 2 in, 2 out]
                    n215 = property on="Capacitance [pF]" class="WFGraph (strict)"("XScale.Maximum"=w316) -> ()  [unwired: 2 in, 2 out]
                    n216 = property on="Defects" class="IntGraph (strict)"("XScale.Maximum"=w316) -> ()  [unwired: 2 in, 2 out]
                    n217 = property on="Resistance [MW]" class="WFGraph (strict)"("XScale.Maximum"=w316) -> ()  [unwired: 2 in, 2 out]
                    n218 = property on="Capacitance [pF]" class="WFGraph (strict)"("XScale.Minimum"=w318) -> ()  [unwired: 2 in, 2 out]
                    n219 = property on="Defects" class="IntGraph (strict)"("XScale.Minimum"=w318) -> ()  [unwired: 2 in, 2 out]
                    n220 = property on="Current [nA]" class="WFGraph (strict)"("XScale.Minimum"=w318) -> ()  [unwired: 2 in, 2 out]
                    n221 = property on="Resistance [MW]" class="WFGraph (strict)"("XScale.Minimum"=w318) -> ()  [unwired: 2 in, 2 out]
                    n222 = call "DefectArrays.vi"("action"=w322, "Region Index"=w320) -> ("Defect array OUT"=w321:i32[][])  [unwired: 1 in, 7 out]
                    n223 = local write "Defects"(w321) -> ()
                  }
                }
                n224 = call "MultiRegionData.vi"("Action"=T5."Reset", "Array Size / Index"=0, "Region index"=w306) -> ()  [unwired: 3 in, 2 out]
                n225 = Bundle(cluster=cluster{string, i32} {"", 0}, w307, w306) -> (w305:cluster{string, i32})
                n226 = Build Array (concatenate)(w314, w305) -> (w313:cluster{string, i32}[])
              }
            }
            n227 = Add(x=w295, y=w290) -> (x+y=w293:i32)
          }
          "total strip number" <- w283
          n228 = property on="Show:" class="Ring (strict)"("StringsAndValues[]"=w284) -> ()  [unwired: 2 in, 2 out]
        }
        frame #2 {
          n229 = case shown="False" w323 {
            frame False {
              n230 = global read "QC_MeasurementSetup.vi" "Striptest Measurement Parameters"() -> (w352:T8)
              n231 = Unbundle By Name(w352) -> ("LCR"=w329:refnum<class "LCRControl.lvclass">, "SMU"=w330:refnum<class "SupplyControl.lvclass">, "Bias Supply"=w331:refnum<class "SupplyControl.lvclass">, "Bias Voltage [V]"=w341:dbl, "Measurement switch"=w326:refnum<class "Switching.lvclass">, "ProbeStation"=w328:refnum<class "ProbeStationControl.lvclass">, "Probe Card Channels"=w325:i32, "Single Needle"=w324:bool)
              n232 = call-dynamic "Supply_Reset.vi"("SupplyControl in"=w331) -> ("error out"=w345:errorcluster, "SupplyControl out"=w348:refnum<class "SupplyControl.lvclass">)  [unwired: 9 in]
              n233 = call-dynamic "Supply_Init.vi"("error in (no error)"=w345, "SupplyControl in"=w348) -> ("error out"=w346:errorcluster, "SupplyControl out"=w347:refnum<class "SupplyControl.lvclass">)  [unwired: 8 in]
              n234 = call-dynamic "Supply_Arm.vi"("error in (no error)"=w346, "SupplyControl in"=w347) -> ("error out"=w343:errorcluster, "SupplyControl out"=w344:refnum<class "SupplyControl.lvclass">)  [unwired: 8 in]
              n235 = call "SupplyRamp.vi"("error in"=w343, "Requested Voltage"=w341, "Step Size"=10.0, "Step Delay"=1000, "Supply IN"=w344, "Starting Voltage"=0.0) -> ("error out"=w342:errorcluster, "Supply OUT"=w327:refnum<class "SupplyControl.lvclass">, "Compliance exceeded"=w335:bool, "Current Voltage"=→"Current Bias Voltage [V]":dbl)  [unwired: 2 in]
              n236 = call-dynamic "Supply_Reset.vi"("error in (no error)"=w342, "SupplyControl in"=w330) -> ("error out"=w339:errorcluster, "SupplyControl out"=w338:refnum<class "SupplyControl.lvclass">)  [unwired: 8 in]
              n237 = call-dynamic "Supply_Init.vi"("error in (no error)"=w339, "SupplyControl in"=w338) -> ("error out"=w340:errorcluster, "SupplyControl out"=w337:refnum<class "SupplyControl.lvclass">)  [unwired: 8 in]
              n238 = call-dynamic "Supply_Arm.vi"("error in (no error)"=w340, "SupplyControl in"=w337) -> ("error out"=w353:errorcluster)  [unwired: 8 in, 1 out]
              n239 = call-dynamic "MatrixSwitch.vi"("error in (no error)"=w353, "Action"=T6."Reset", "Switching in"=w326) -> ("error out"=w332:errorcluster, "Switching out"=w333:refnum<class "Switching.lvclass">)  [unwired: 6 in, 1 out]
              n240 = case shown="False" w335 {
                selector: w335 -> [_ w441]
                tunnel: w333 -> [w383 _]
                tunnel: w332 -> [w382 _]
                tunnel: w329 -> [w381 _]
                tunnel: w328 -> [w380 _]
                tunnel: w327 -> [w379 _]
                tunnel: w325 -> [w378 _]
                tunnel: w324 -> [w377 _]
                frame False {
                  n241 = flat-sequence {
                    tunnel: w383 -> [w389]
                    tunnel: [w389] -> w376
                    tunnel: w382 -> [w392]
                    tunnel: w381 -> [w388]
                    tunnel: [w388] -> w375
                    tunnel: w380 -> [w390]
                    tunnel: w379 -> [w387]
                    tunnel: [w387] -> w374
                    tunnel: w378 -> [w386]
                    tunnel: [w386] -> w373
                    tunnel: w377 -> [w385]
                    tunnel: [w385] -> w372
                    tunnel: [w391] -> w371
                    tunnel: w376 -> [w396]
                    tunnel: [w396] -> w359
                    tunnel: w375 -> [w402]
                    tunnel: [w402] -> w358
                    tunnel: w374 -> [w397]
                    tunnel: [w397] -> w357
                    tunnel: w373 -> [w395]
                    tunnel: [w395] -> w356
                    tunnel: w372 -> [w394]
                    tunnel: [w394] -> w355
                    tunnel: w371 -> [w399]
                    tunnel: [w403] -> w354
                    tunnel: w359 -> [w407]
                    tunnel: [w407] -> w370
                    tunnel: w358 -> [w405]
                    tunnel: [w405] -> w369
                    tunnel: w357 -> [w404]
                    tunnel: [w404] -> w368
                    tunnel: w356 -> [w408]
                    tunnel: [w408] -> w367
                    tunnel: w355 -> [w409]
                    tunnel: [w409] -> w366
                    tunnel: w354 -> [w410]
                    tunnel: [w411] -> w365
                    tunnel: w370 -> [w419]
                    tunnel: [w419] -> w364
                    tunnel: w369 -> [w421]
                    tunnel: w368 -> [w418]
                    tunnel: [w418] -> w363
                    tunnel: w367 -> [w417]
                    tunnel: [w417] -> w362
                    tunnel: w366 -> [w416]
                    tunnel: [w416] -> w361
                    tunnel: w365 -> [w422]
                    tunnel: [w420] -> w360
                    tunnel: w364 -> [w428]
                    tunnel: w363 -> [w429]
                    tunnel: w362 -> [w424]
                    tunnel: w361 -> [w423]
                    tunnel: w360 -> [w427]
                    frame #0 {
                      n242 = call-dynamic "Prober_ChuckUpDown.vi"("error in (no error)"=w392, "Direction"=enum16{"up", "down"}."down", "ProbeStationControl in"=w390) -> ("error out"=w391:errorcluster)  [unwired: 6 in, 2 out]
                    }
                    frame #1 {
                      n243 = local write "Status:"("Trimming LCR ..." ("STATUS 1")) -> ()
                      n244 = call-dynamic "Supply_ZeroCheck.vi"("error in (no error)"=w399, "enable/disable"=TRUE, "SupplyControl in"=w397) -> ("error out"=w398:errorcluster)  [unwired: 7 in, 1 out]
                      n245 = call-dynamic "LCR_Init.vi"("error in (no error)"=w398, "LCRControl in"=w402) -> ("error out"=w403:errorcluster)  [unwired: 8 in, 1 out]
                    }
                    frame #2 {
                      n246 = Wait (ms)(milliseconds to wait=1000) -> ()  [unwired: 1 out]
                      n247 = call-dynamic "MuxCardSwitch.vi"("Single Needle"=w409, "Probe Card Channels"=w408, "error in (no error)"=w410, "Switch to channel"=1, "Switching in"=w407) -> ("error out"=w412:errorcluster, "Switching out"=w406:refnum<class "Switching.lvclass">)  [unwired: 4 in, 1 out]
                      n248 = call-dynamic "MatrixSwitch.vi"("error in (no error)"=w412, "Action"=T6."Striptest LCR", "Switching in"=w406) -> ("error out"=w411:errorcluster)  [unwired: 6 in, 2 out]
                    }
                    frame #3 {
                      n249 = call-dynamic "LCR_TrimOC.vi"("error in (no error)"=w422, "LCRControl in"=w421) -> ("error out"=w420:errorcluster)  [unwired: 8 in, 1 out]
                    }
                    frame #4 {
                      w435 = u16 0 items=["Open", "Close"] ("Switch action")
                      n250 = call-dynamic "Supply_ZeroCheck.vi"("error in (no error)"=w427, "enable/disable"=TRUE, "SupplyControl in"=w429) -> ("error out"=w426:errorcluster)  [unwired: 7 in, 1 out]
                      n251 = call-dynamic "MatrixSwitchSingle.vi"("Switch action"=w435, "error in (no error)"=w426, "Matrix Y"=1, "Matrix X"=3, "Switching in"=w428) -> ("error out"=w431:errorcluster, "Switching out"=w432:refnum<class "Switching.lvclass">)  [unwired: 4 in, 1 out]
                      n252 = call-dynamic "MatrixSwitchSingle.vi"("Switch action"=w435, "error in (no error)"=w431, "Matrix Y"=2, "Matrix X"=4, "Switching in"=w432) -> ("error out"=w430:errorcluster, "Switching out"=w425:refnum<class "Switching.lvclass">)  [unwired: 4 in, 1 out]
                      n253 = call-dynamic "MuxCardSwitch.vi"("Single Needle"=w423, "Probe Card Channels"=w424, "error in (no error)"=w430, "Switch to channel"=-1, "Switching in"=w425) -> ()  [unwired: 4 in, 3 out]
                    }
                  }
                  n254 = local write "Bias On/Off:"(TRUE ("Bias On?")) -> ()
                }
                frame True {
                  n255 = property on="Bias On/Off:" class="Bool (strict)"("Blinking"=w441) -> ()  [unwired: 2 in, 2 out]
                  n256 = local write "Status:"("Compliance exceeded\nRUN ABORTED") -> ()
                }
              }
            }
            frame True {
            }
          }
        }
        frame #3 {
          n257 = property on="Bias On/Off:" class="Bool (strict)"() -> ("Blinking"=w443:bool)  [unwired: 2 in, 2 out]
          n258 = case shown="False" w443 {
            tunnel: w444 -> [w448 _]
            tunnel: w442 -> [w445 _]
            frame False {
              w449 = 0
              n259 = property on="Abort" class="Bool (strict)"("DisabledEnum"=w449) -> ()  [unwired: 2 in, 2 out]
              n260 = property on="Auto ReCheck" class="Bool (strict)"("DisabledEnum"=w449) -> ()  [unwired: 2 in, 2 out]
              n261 = local read "Single Needle"() -> (w447:bool)
              n262 = Or(x=w447, y=w448) -> (x .or. y?=w446:bool)
              n263 = case shown="False" w446 {
                tunnel: [w452 FALSE] -> w450
                tunnel: w445 -> [w451 _]
                frame False {
                  n264 = stacked-sequence {
                    tunnel: [_ w461] -> w452
                    tunnel: w451 -> [_ _]
                    frame #0 {
                      n265 = local write "Status:"("Reference measurement") -> ()
                      n266 = global read "QC_MeasurementSetup.vi" "Striptest Measurement Parameters"() -> (w453:T8)
                      n267 = Unbundle By Name(w453) -> ("Measurement switch"=w454:refnum<class "Switching.lvclass">)
                      n268 = call-dynamic "MatrixSwitch.vi"("Action"=T6."Striptest SMU", "Switching in"=w454) -> ()  [unwired: 7 in, 3 out]
                    }
                    frame #1 {
                      n269 = local read "settling\ndelay [ms]"() -> (w460:i32)
                      n270 = call "CurrentCorrection.vi"("Action"=T7."Reference measurement", "settling\ndelay"=w460) -> ("Compliance exceeded?"=w461:bool, "Current Reference 100V"=→"Current Reference 100V":dbl[], "Current Reference 10V"=→"Current Reference 10V":dbl[])  [unwired: 3 in, 2 out]
                    }
                  }
                }
                frame True {
                }
              }
              n271 = case shown="False" w450 {
                frame False {
                  n272 = local write "Status:"("RUN IN PROGRESS" ("STATUS 1")) -> ()
                }
                frame True {
                  n273 = property on="Bias On/Off:" class="Bool (strict)"("Blinking"=TRUE ("Compliance?")) -> ()  [unwired: 2 in, 2 out]
                  n274 = local write "Status:"("Compliance exceeded\nRUN ABORTED") -> ()
                }
              }
            }
            frame True {
            }
          }
        }
        frame #4 {
          n275 = property on="Bias On/Off:" class="Bool (strict)"() -> ("Blinking"=w468:bool)  [unwired: 2 in, 2 out]
          n276 = case shown="False" w468 {
            tunnel: w469 -> [w479 _]
            tunnel: w467 -> [w478 _]
            tunnel: w466 -> [w477 _]
            frame False {
              n277 = Array Size(array=w479) -> (size(s)=w480:i32)
              n278 = local read "Temperature Progression"() -> (w471:T3)
              n279 = local read "probe points per region"() -> (w472:i32[])
              n280 = local read "max scale array"() -> (w475:i32[])
              n281 = local read "min scale array"() -> (w474:i32[])
              n282 = for {
                N: w480 -> [_]
                tunnel: w479 -> [w493] mode=indexing
                tunnel: w478 -> [w492] mode=indexing
                tunnel: w477 -> [w491]
                shift-right: [w485] -> _
                shift-left: 0 -> [w490]
                tunnel: w475 -> [w488] mode=indexing
                tunnel: w474 -> [w489] mode=indexing
                shift-right: [w484] -> _
                shift-left: 0 -> [w486]
                tunnel: w472 -> [w483] mode=indexing
                shift-right: [w481] -> w470
                shift-left: w471 -> [w482]
                i -> [w487]
                n283 = case shown="True" w493 {
                  tunnel: w492 -> [_ w509]
                  tunnel: w491 -> [_ _]
                  tunnel: w490 -> [w495 w510]
                  tunnel: w489 -> [_ w505]
                  tunnel: w488 -> [_ w502]
                  tunnel: w487 -> [_ w507]
                  tunnel: w486 -> [w497 w504]
                  tunnel: [w494 w503] -> w485
                  tunnel: [w497 w501] -> w484
                  tunnel: w483 -> [_ w500]
                  tunnel: w482 -> [w496 w499]
                  tunnel: [w496 w498] -> w481
                  frame False {
                    n284 = Increment(x=w495) -> (x+1=w494:i32)
                  }
                  frame True {
                    n285 = local write "Show:"(w510) -> ()
                    n286 = Unbundle By Name(w509) -> ("Region"=→"Probing Region:":string, "ProbePoints"=w506:T14)
                    n287 = while {
                      tunnel: w507 -> [w511]
                      tunnel: w506 -> [w531]
                      shift-right: [w524] -> _
                      shift-left: w505 -> [w513]
                      shift-right: [w525] -> w501
                      shift-left: w504 -> [w526]
                      tunnel: w502 -> [w523]
                      tunnel: w500 -> [_]
                      shift-right: [w521] -> w498
                      shift-left: w499 -> [w522]
                      i -> [w527]
                      stop <- w530 stop-if-true
                      n288 = Index Array(array=w531, index=w513) -> (element=w532:T15)
                      n289 = Equal To 0?(x=w526) -> (x = 0?=w533:bool)
                      n290 = Equal?(x=w513, y=w523) -> (x = y?=w512:bool)
                      n291 = case shown="True" w533 {
                        frame False {
                        }
                        frame True {
                          n292 = local read "Probe Card Channels"() -> (w1069:i32)
                          n293 = local read "total strip number"() -> (w1070:u32)
                          n294 = Divide(x=w1070, y=w1069) -> (x/y=w1068:dbl)
                          n295 = To Long Integer(number=w1068) -> (32bit integer=w1067:i32)
                          n296 = call "RunTime.vi"("no. measurements"=w1067, "Flag"=1) -> ()  [unwired: 2 in, 4 out]
                        }
                      }
                      n297 = case shown="True" w512 {
                        tunnel: w511 -> [_ w534]
                        frame False {
                        }
                        frame True {
                          n298 = stacked-sequence {
                            tunnel: w534 -> [_ w537 w542]
                            frame #0 {
                              n299 = Wait (ms)(milliseconds to wait=100) -> ()  [unwired: 1 out]
                            }
                            frame #1 {
                              n300 = Increment(x=w537) -> (x+1=w540:i32)
                              n301 = Multiply(x=w540, y=111) -> (x*y=w538:i32)
                              n302 = call "SaveJPEG.vi"("Picture No."=w538, "Test"="Striptest") -> ()  [unwired: 1 in, 2 out]
                            }
                            frame #2 {
                              n303 = local read "probe points per region"() -> (w544:i32[])
                              n304 = Index Array(array=w544, index=w542) -> ()  [unwired: 1 out]
                              n305 = local read "Probing Region:"() -> (w541:string)
                              n306 = call "SaveStriptestRecoveryFiles.vi"("Array Titles"="ProbeplanIndex Current PinholeFlag Capacitance Resistance", "Strip Segment"=w541, "Region #"=w542) -> ()  [unwired: 3 in, 2 out]
                            }
                          }
                        }
                      }
                      n307 = Unbundle By Name(w532) -> ("CardViable?"=w518:bool)
                      n308 = property on="Bias On/Off:" class="Bool (strict)"() -> ("Blinking"=w528:bool)  [unwired: 2 in, 2 out]
                      n309 = property on="Bias On/Off:" class="Bool (strict)"() -> ("Blinking"=w520:bool)  [unwired: 2 in, 2 out]
                      n310 = local read "Abort"() -> (w516:bool)
                      n311 = Not(x=w520) -> (.not. x?=w519:bool)
                      n312 = Not(x=w516) -> (.not. x?=w515:bool)
                      n313 = Compound Arithmetic op=AND(w518, w519, w515) -> (w517:bool)
                      n314 = Build Array(w528, "Abort", w512) -> (w529:bool[])
                      n315 = Or Array Elements(Boolean array=w529) -> (logical OR=w530:bool)
                      n316 = case shown="True" w517 {
                        tunnel: w511 -> [_ w562]
                        tunnel: w531 -> [_ w561]
                        tunnel: w513 -> [w545 w556]
                        tunnel: w527 -> [_ w560]
                        tunnel: w526 -> [w548 w559]
                        tunnel: [w548 w558] -> w525
                        tunnel: [w546 w557] -> w524
                        tunnel: w522 -> [w547 w555]
                        tunnel: [w547 w554] -> w521
                        frame False {
                          n317 = Increment(x=w545) -> (x+1=w546:i32)
                        }
                        frame True {
                          n318 = global read "QC_MeasurementSetup.vi" "Striptest Measurement Parameters"() -> (w552:T8)
                          n319 = Unbundle By Name(w552) -> ("ProbeStation"=w551:refnum<class "ProbeStationControl.lvclass">, "Measurement switch"=w553:refnum<class "Switching.lvclass">, "Temperature Readout"=w549:enum16{"Read Arduino", "Enter manually"}, "Arduino"=w550:refnum<class "ArduinoControl.lvclass">)
                          n320 = stacked-sequence {
                            tunnel: w562 -> [w576 w857 w945 w1037 _]
                            tunnel: w561 -> [w566 _ _ _ _]
                            tunnel: w556 -> [w565 _ _ _ w1057]
                            tunnel: w559 -> [_ _ _ _ w1066]
                            tunnel: w560 -> [_ w856 w944 w1036 w1055]
                            tunnel: [_ _ _ _ w1058] -> w558
                            tunnel: [_ _ _ _ w1065] -> w557
                            tunnel: w555 -> [_ w851 _ _ _]
                            tunnel: [_ w850 _ _ _] -> w554
                            tunnel: w553 -> [_ w854 w942 _ _]
                            tunnel: w551 -> [w564 _ _ _ _]
                            tunnel: w550 -> [_ w853 _ _ _]
                            tunnel: w549 -> [_ w852 _ _ _]
                            frame #0 {
                              # "If probepoint label defined as Strip or Channel, use\nthat as the channel number in the data array."
                              n321 = local write "disabled channels"(i32[] []) -> ()
                              n322 = Index Array(array=w566, index=w565) -> (element=w583:T15)
                              n323 = Unbundle(w583) -> ("Label"=w579:string)  [unwired: 3 out]
                              "Probe Point:" <- w579
                              n324 = local read "Simulation?"() -> (w570:bool)
                              n325 = local read "Abort"() -> (w572:bool)
                              n326 = Format Into String(format string="Moving to %s", w579) -> (resulting string=w582:string)  [unwired: 2 in, 1 out]
                              n327 = local write "Status:"(w582) -> ()
                              n328 = local read "Probe Card Channels"() -> (w573:i32)
                              n329 = Or(x=w572, y=w570) -> (x .or. y?=w571:bool)
                              n330 = case shown="False" w571 {
                                tunnel: w576 -> [w842 _]
                                tunnel: w565 -> [w843 _]
                                tunnel: w573 -> [w844 _]
                                tunnel: w564 -> [w840 _]
                                frame False {
                                # "Move to Strip"
                                n331 = local read "Single Needle"() -> (w846:bool)
                                n332 = call "MoveToStrip.vi"("Single Needle"=w846, "Strip No."=w843, "Region"=w842, "ProbeStationControl in"=w840) -> ("Z [µm]"=w841:i32)  [unwired: 5 in, 2 out]
                                n333 = local read "Z profile"() -> (w849:i32[][])
                                n334 = Initialize Array(w841, w844, 1) -> (w847:i32[][])
                                n335 = Replace Array Subset(array=w849, new element=w847, index (row)=w843, index (col)=w842) -> (w848:i32[][])
                                n336 = local write "Z profile"(w848) -> ()
                                }
                                frame True {
                                }
                              }
                              n337 = xnode "Match Regular Expression"("input string"=w579, "regular expression"="(Strip|Channel)\\s+(\\d+)", "ignore case? (F)"=TRUE) -> ("submatch 2"=w569:string)  [unwired: 3 in, 6 out]
                              n338 = Empty String/Path?(string/path=w569) -> (empty?=w568:bool)
                              n339 = Not(x=w568) -> (.not. x?=w567:bool)
                              n340 = case shown="True" w567 {
                                tunnel: [w585 w595] -> w577
                                tunnel: w565 -> [w587 w593]
                                tunnel: w573 -> [w586 w594]
                                tunnel: w566 -> [_ w592]
                                frame False {
                                n341 = for {
                                N: w586 -> [_]
                                tunnel: w587 -> [w590]
                                tunnel: [w588] -> w585 mode=indexing
                                i -> [w591]
                                # "Actually use the probepoint\nindex"
                                n342 = Add(x=w590, y=w591) -> (x+y=w589:i32)
                                n343 = Increment(x=w589) -> (x+1=w588:i32)
                                }
                                }
                                frame True {
                                n344 = for {
                                N: w594 -> [_]
                                tunnel: [w604] -> w595 mode=indexing
                                tunnel: w593 -> [w601]
                                tunnel: w592 -> [w599]
                                i -> [w602]
                                n345 = Add(x=w601, y=w602) -> (x+y=w600:i32)
                                n346 = Index Array(array=w599, index=w600) -> (element=w598:T15)
                                n347 = Unbundle By Name(w598) -> ("Label"=w597:string)
                                n348 = xnode "Match Regular Expression"("input string"=w597, "regular expression"="(Strip|Channel)\\s+(\\d+)") -> ("submatch 2"=w596:string)  [unwired: 4 in, 6 out]
                                n349 = Scan From String(format string="%d", input string=w596) -> (output 1=w604:i32)  [unwired: 3 in, 3 out]
                                }
                                }
                              }
                              n350 = To Double Precision Float(number=w577) -> (double precision float=w574:dbl[])
                              n351 = call "MultiRegionData.vi"("Action"=T5."Add Array", "Array No."=0 ("Array Size / Index"), "Array IN"=w574, "Region index"=w576) -> ()  [unwired: 2 in, 2 out]
                            }
                            frame #1 {
                              # "Pinholes"
                              n352 = local read "Simulation?"() -> (w855:bool)
                              n353 = stacked-sequence {
                                tunnel: w855 -> [w873 w894]
                                tunnel: w857 -> [_ w896]
                                tunnel: w856 -> [_ w895]
                                tunnel: w854 -> [w872 _]
                                tunnel: w853 -> [w870 _]
                                tunnel: w852 -> [w871 _]
                                tunnel: w851 -> [w864 _]
                                tunnel: [w862 _] -> w850
                                frame #0 {
                                n354 = Unbundle By Name(w864) -> ("Time Array"=w866:string[], "Temperature Array [°C]"=w861:dbl[], "Humidity Array [RH %]"=w860:dbl[])
                                n355 = case shown="\"Read Arduino\", Default" w871 {
                                tunnel: w870 -> [w881 _]
                                tunnel: [w880 _] -> w869
                                tunnel: w861 -> [w876 w885]
                                tunnel: w860 -> [w877 w887]
                                tunnel: [w875 w884] -> w859
                                tunnel: [w874 w883] -> w858
                                frame "Read Arduino", Default {
                                n356 = call "ArduinoRead.vi"("Arduino function"=enum16{"T/RH", "Interlock", "Edgesense"}."T/RH", "ArduinoControl in"=w881) -> ("error out"=w880:errorcluster, "rel. Humidity [%]"=w878:dbl, "Temperature [°C]"=w879:dbl)  [unwired: 4 in, 3 out]
                                n357 = Build Array (concatenate)(w876, w879) -> (w875:dbl[])
                                n358 = Build Array (concatenate)(w877, w878) -> (w874:dbl[])
                                }
                                frame "Enter manually" {
                                n359 = Index Array(array=w885, index=0) -> (element=w886:dbl)
                                n360 = Index Array(array=w887, index=0) -> (element=w888:dbl)
                                n361 = Build Array (concatenate)(w885, w886) -> (w884:dbl[])
                                n362 = Build Array (concatenate)(w887, w888) -> (w883:dbl[])
                                }
                                }
                                n363 = call "RunTime.vi"("Probing done - new estimation"=FALSE, "Flag"=0) -> ("Time so far"=w865:string)  [unwired: 2 in, 3 out]
                                n364 = Build Array (concatenate)(w866, w865) -> (w863:string[])
                                n365 = case shown="False" w873 {
                                tunnel: w872 -> [w893 _]
                                tunnel: w869 -> [w892 _]
                                frame False {
                                n366 = call-dynamic "MatrixSwitch.vi"("error in (no error)"=w892, "Action"=T6."Striptest SMU", "Switching in"=w893) -> ()  [unwired: 6 in, 3 out]
                                }
                                frame True {
                                }
                                }
                                n367 = Bundle By Name(cluster=w864, "Time Array"=w863, "Temperature Array [°C]"=w859, "Humidity Array [RH %]"=w858) -> (w862:T3)
                                }
                                frame #1 {
                                n368 = local read "Abort"() -> (w897:bool)
                                n369 = case shown="False" w897 {
                                tunnel: w896 -> [w905 _]
                                tunnel: w895 -> [_ _]
                                tunnel: w894 -> [w899 _]
                                frame False {
                                w898 = T5."Add Array" ("Action")
                                n370 = case shown="False" w899 {
                                tunnel: [w917 w930] -> w900
                                tunnel: [w914 w929] -> w904
                                frame False {
                                n371 = local read "Thresholds:"() -> (w916:T2)
                                n372 = Unbundle By Name(w916) -> ("Current [nA]"=w915:dbl)
                                n373 = case shown="False" "Rolling\nCurrent Readout" {
                                tunnel: [w922 w924] -> w917
                                tunnel: w915 -> [w918 w927]
                                tunnel: [w921 w926] -> w914
                                tunnel: [w920 w925] -> w913
                                tunnel: "settling\ndelay [ms]" -> [w919 w923]
                                frame False {
                                n374 = call "Pinholes.vi"("Current Threshold [nA]"=w918, "settling\ndelay"=w919) -> ("excluded channels"=w920:i32[], "Current [nA]"=w922:dbl[], "Flag"=w921:i32[])  [unwired: 3 in]
                                }
                                frame True {
                                n375 = call "PinholesRolling.vi"("Current Threshold [nA]"=w927, "settling\ndelay"=w923) -> ("excluded channels"=w925:i32[], "Current [nA]"=w924:dbl[], "Flag"=w926:i32[])  [unwired: 3 in]
                                }
                                }
                                "disabled channels" <- w913
                                }
                                frame True {
                                n376 = local read "Probe Card Channels"() -> (w928:i32)
                                n377 = for {
                                N: w928 -> [_]
                                tunnel: [w932] -> w930 mode=indexing
                                tunnel: [w931] -> w929 mode=indexing
                                # "Simulate"
                                n378 = Random Number (0-1)() -> (number: 0 to 1=w935:dbl)
                                n379 = Greater?(x=w935, y=0.95) -> (0:w936:bool)
                                n380 = case shown="False" w936 {
                                tunnel: [w940 5000.0] -> w932
                                tunnel: w935 -> [w940 _]
                                frame False {
                                }
                                frame True {
                                }
                                }
                                n381 = Greater?(x=w932, y=50.0) -> (0:w933:bool)
                                n382 = case shown="False" w933 {
                                tunnel: [0 1] -> w931
                                frame False {
                                }
                                frame True {
                                }
                                }
                                }
                                }
                                }
                                n383 = Get Date/Time String(want seconds? (F)=TRUE) -> (time string=→"Last Probe at:":string)  [unwired: 2 in, 1 out]
                                n384 = local write "Status:"("Measuring Ipinhole") -> ()
                                n385 = To Double Precision Float(number=w904) -> (double precision float=w903:dbl[])
                                n386 = Index Array(array=w900, index=0) -> (element=→"Current [nA]:":dbl)
                                n387 = call "MultiRegionData.vi"("Action"=w898, "Array No."=1, "Array IN"=w900, "Region index"=w905) -> ()  [unwired: 2 in, 2 out]
                                n388 = call "MultiRegionData.vi"("Action"=w898, "Array No."=2, "Array IN"=w903, "Region index"=w905) -> ()  [unwired: 2 in, 2 out]
                                }
                                frame True {
                                }
                                }
                                }
                              }
                            }
                            frame #2 {
                              # "Capacitance and Resistance"
                              n389 = local read "Simulation?"() -> (w943:bool)
                              n390 = stacked-sequence {
                                seq-local: [_ _ w958 _] -> [_ _ _ w1016]
                                tunnel: w945 -> [_ _ w965 _]
                                tunnel: w944 -> [_ _ _ _]
                                tunnel: w943 -> [w947 w951 w957 w1015]
                                tunnel: w942 -> [w946 w950 w956 w1014]
                                frame #0 {
                                n391 = case shown="False" w947 {
                                tunnel: w946 -> [w948 _]
                                frame False {
                                n392 = call-dynamic "MatrixSwitch.vi"("Action"=T6."Ground", "Switching in"=w948) -> ()  [unwired: 7 in, 3 out]
                                }
                                frame True {
                                }
                                }
                                }
                                frame #1 {
                                n393 = case shown="False" w951 {
                                tunnel: w950 -> [w953 _]
                                frame False {
                                n394 = call-dynamic "MatrixSwitch.vi"("Action"=T6."Striptest LCR", "Switching in"=w953) -> ()  [unwired: 7 in, 3 out]
                                }
                                frame True {
                                }
                                }
                                n395 = local write "Status:"("Measuring capacitance..." ("STATUS 1")) -> ()
                                }
                                frame #2 {
                                w955 = T5."Add Array" ("Action")
                                w961 = 0
                                n396 = local read "Probe Card Channels"() -> (w958:i32)
                                n397 = local read "disabled channels"() -> (w960:i32[])
                                n398 = for {
                                N: w958 -> [_]
                                tunnel: [w974] -> w959 mode=indexing
                                tunnel: [w973] -> w962 mode=indexing
                                tunnel: w960 -> [w970]
                                tunnel: w958 -> [w972]
                                tunnel: w957 -> [w969]
                                tunnel: w956 -> [w968]
                                i -> [w971]
                                n399 = case shown="False" w969 {
                                tunnel: [w983 w1005] -> w974
                                tunnel: [w982 w1004] -> w973
                                tunnel: w972 -> [w979 _]
                                tunnel: w971 -> [w977 _]
                                tunnel: w970 -> [w978 _]
                                tunnel: w968 -> [w975 _]
                                frame False {
                                n400 = Increment(x=w977) -> (x+1=w976:i32)
                                n401 = Search 1D Array(1D array=w978, element=w976) -> (index of element=w981:i32)  [unwired: 1 in]
                                n402 = Less Than 0?(x=w981) -> (x < 0?=w980:bool)
                                n403 = case shown="True" w980 {
                                tunnel: [w986 w992] -> w983
                                tunnel: [w984 w991] -> w982
                                tunnel: w979 -> [_ w990]
                                tunnel: w976 -> [_ w989]
                                tunnel: w978 -> [_ w988]
                                tunnel: w975 -> [_ w987]
                                frame False {
                                w986 = -1.0
                                n404 = Divide(x=w986, y=1000000.0) -> (x/y=w984:dbl)
                                }
                                frame True {
                                n405 = stacked-sequence {
                                tunnel: w990 -> [w995 _ _]
                                tunnel: w989 -> [w997 _ _]
                                tunnel: w988 -> [w996 _ _]
                                tunnel: [_ _ w1003] -> w992
                                tunnel: [_ _ w1002] -> w991
                                tunnel: w987 -> [w994 _ _]
                                frame #0 {
                                n406 = local read "Single Needle"() -> (w993:bool)
                                n407 = call-dynamic "MuxCardSwitch.vi"("Single Needle"=w993, "Probe Card Channels"=w995, "disabled channels"=w996, "Switch to channel"=w997, "Switching in"=w994) -> ()  [unwired: 4 in, 3 out]
                                }
                                frame #1 {
                                n408 = local read "settling\ndelay [ms]"() -> (w998:i32)
                                n409 = Wait (ms)(milliseconds to wait=w998) -> ()  [unwired: 1 out]
                                }
                                frame #2 {
                                n410 = global read "QC_MeasurementSetup.vi" "Striptest Measurement Parameters"() -> (w1001:T8)
                                n411 = Unbundle By Name(w1001) -> ("LCR"=w1000:refnum<class "LCRControl.lvclass">, "AC frequency [Hz]"=w999:i32)
                                n412 = call-dynamic "LCR_Readout.vi"("Frequency in Hz"=w999, "LCRControl in"=w1000) -> ("Resistance in Ohm"=w1002:dbl, "Capacitance in pF"=w1003:dbl)  [unwired: 6 in, 2 out]
                                }
                                }
                                }
                                }
                                }
                                frame True {
                                n413 = Random Number (0-1)() -> (number: 0 to 1=w1009:dbl)
                                n414 = Random Number (0-1)() -> (number: 0 to 1=w1013:dbl)
                                n415 = Multiply(x=w1013, y=18.0) -> (x*y=w1011:dbl)
                                n416 = Multiply(x=w1009, y=0.6) -> (x*y=w1006:dbl)
                                n417 = Add(x=w1011, y=64.0) -> (x+y=w1005:dbl)
                                n418 = Add(x=1.5 ("Resistance"), y=w1006) -> (x+y=w1004:dbl)
                                }
                                }
                                }
                                n419 = Index Array(array=w962, index=w961) -> (element=→"Reistance [MW]:":dbl)
                                n420 = Index Array(array=w959, index=w961) -> (element=→"Capacitance [pF]:":dbl)
                                n421 = call "MultiRegionData.vi"("Action"=w955, "Array No."=3, "Array IN"=w959, "Region index"=w965) -> ()  [unwired: 2 in, 2 out]
                                n422 = call "MultiRegionData.vi"("Action"=w955, "Array No."=4, "Array IN"=w962, "Region index"=w965) -> ()  [unwired: 2 in, 2 out]
                                }
                                frame #3 {
                                n423 = case shown="False" w1015 {
                                tunnel: w1016 -> [w1019 _]
                                tunnel: w1014 -> [w1017 _]
                                frame False {
                                n424 = local read "Single Needle"() -> (w1018:bool)
                                n425 = call-dynamic "MuxCardSwitch.vi"("Single Needle"=w1018, "Probe Card Channels"=w1019, "Switch to channel"=-1, "Switching in"=w1017) -> ()  [unwired: 5 in, 3 out]
                                }
                                frame True {
                                }
                                }
                                }
                              }
                            }
                            frame #3 {
                              # "If selected region is CURRENT region being probed,\nuse number probed so far\notherwise total number of probepoints in this region"
                              n426 = local read "Region Indices"() -> (w1039:i32[])
                              n427 = Index Array(array=w1039, index="Show:") -> (element=w1035:i32)
                              n428 = Equal?(x=w1035, y=w1037) -> (x = y?=w1038:bool)
                              n429 = case shown="True" w1038 {
                                tunnel: w1036 -> [_ w1051]
                                tunnel: [w1047 w1050] -> w1034
                                tunnel: w1035 -> [w1046 _]
                                frame False {
                                n430 = local read "probe points per region"() -> (w1048:i32[])
                                n431 = Index Array(array=w1048, index=w1046) -> (element=w1047:i32)
                                }
                                frame True {
                                n432 = local read "Probe Card Channels"() -> (w1049:i32)
                                n433 = Add(x=w1049, y=w1051) -> (x+y=w1050:i32)
                                }
                              }
                              n434 = local read "max scale array"() -> (w1031:i32[])
                              n435 = local read "min scale array"() -> (w1033:i32[])
                              n436 = local read "Thresholds:"() -> (w1045:T2)
                              n437 = Index Array(array=w1031, index="Show:") -> (element=w1028:i32)
                              n438 = Index Array(array=w1033, index="Show:") -> (element=w1030:i32)
                              n439 = call "DisplayStriptestData.vi"("min scale array"=w1033, "max scale array"=w1031, "# probed"=w1034, "Display Stats?"=TRUE, "Thresholds"=w1045, "Region"=w1035) -> ("Defects"=→"Defects":i32[][], "Resistance [MW]"=→"Resistance [MW]":cluster{u32, i32, "Array OUT":dbl[]}, "Capacitance [pF]"=→"Capacitance [pF]":cluster{u32, i32, "Array OUT":dbl[]}, "Current [nA]"=→"Current [nA]":cluster{u32, i32, "Array OUT":dbl[]}, "Strip Quality Data"=w1041:T16)
                              n440 = Increment(x=w1028) -> (x+1=w1027:i32)
                              n441 = Increment(x=w1030) -> (x+1=w1029:i32)
                              n442 = property on="Capacitance [pF]" class="WFGraph (strict)"("XScale.Maximum"=w1027) -> ()  [unwired: 2 in, 2 out]
                              n443 = property on="Resistance [MW]" class="WFGraph (strict)"("XScale.Maximum"=w1027) -> ()  [unwired: 2 in, 2 out]
                              n444 = property on="Current [nA]" class="WFGraph (strict)"("XScale.Maximum"=w1027) -> ()  [unwired: 2 in, 2 out]
                              n445 = property on="Capacitance [pF]" class="WFGraph (strict)"("XScale.Minimum"=w1029) -> ()  [unwired: 2 in, 2 out]
                              n446 = property on="Resistance [MW]" class="WFGraph (strict)"("XScale.Minimum"=w1029) -> ()  [unwired: 2 in, 2 out]
                              n447 = property on="Current [nA]" class="WFGraph (strict)"("XScale.Minimum"=w1029) -> ()  [unwired: 2 in, 2 out]
                              n448 = property on="Defects" class="IntGraph (strict)"("XScale.Minimum"=w1029) -> ()  [unwired: 2 in, 2 out]
                              n449 = Increment(x=w1027) -> (x+1=w1026:i32)
                              n450 = property on="Defects" class="IntGraph (strict)"("XScale.Maximum"=w1026) -> ()  [unwired: 2 in, 2 out]
                              n451 = Unbundle By Name(w1041) -> ("pass Rate in %"=→"% OK:":dbl, "Bad channel list"=→"Bad Strip List":i32[], "No of bad strips"=w1024:i32, "Number of defects per category"=→"defect type array":i32[])
                              n452 = local write "# total defects:"(w1024) -> ()
                            }
                            frame #4 {
                              # "save image if required"
                              n453 = Increment(x=w1057) -> (x+1=w1065:i32)
                              n454 = call "RunTime.vi"("Probing done - new estimation"=TRUE, "Flag"=0) -> ("Estimated Completion Time"=w1062:string, "Time so far"=→"Run Duration:":string)  [unwired: 2 in, 2 out]
                              n455 = Scan From String(format string="%s %s", input string=w1062) -> (output 2=→"Estimated Completion:":string)  [unwired: 5 in, 3 out]
                              n456 = local read "Probe Card Channels"() -> (w1056:i32)
                              n457 = Quotient & Remainder(x=w1055, y=w1056) -> (floor(x/y)=w1054:i32)  [unwired: 1 out]
                              n458 = Add(x=w1056, y=w1066) -> (x+y=w1058:i32)
                              n459 = Increment(x=w1054) -> (x+1=w1053:i32)
                              n460 = local write "# probed"(w1058) -> ()
                              n461 = call "SaveJPEG.vi"("Picture No."=w1053, "Test"="Striptest") -> ()  [unwired: 1 in, 2 out]
                            }
                          }
                        }
                      }
                    }
                    n462 = Increment(x=w510) -> (x+1=w503:i32)
                  }
                }
              }
              n463 = local write "Temperature Progression"(w470) -> ()
            }
            frame True {
            }
          }
        }
        frame #5 {
          # "Ramp down volts now"
          n464 = case shown="False" w1073 {
            tunnel: w1072 -> [w1094 _]
            frame False {
              w1099 = "0"
              n465 = property on="Abort" class="Bool (strict)"("DisabledEnum"=2) -> ()  [unwired: 2 in, 2 out]
              n466 = local read "# probed"() -> (w1092:i32)
              n467 = call-dynamic "Prober_ChuckUpDown.vi"("Direction"=enum16{"up", "down"}."down", "ProbeStationControl in"=w1094) -> ("error out"=w1096:errorcluster, "ProbeStationControl out"=w1095:refnum<class "ProbeStationControl.lvclass">)  [unwired: 7 in, 1 out]
              n468 = call "SaveJPEG.vi"("Picture No."=w1092, "Test"="Striptest") -> ()  [unwired: 1 in, 2 out]
              n469 = call-dynamic "Prober_MoveToXYZTheta.vi"("Theta location [mdeg]"="none", "ProbeStationControl in"=w1095, "error in (no error)"=w1096, "Z location [µm]"="down", "Y location [µm]"=w1099, "X location [µm]"=w1099) -> ()  [unwired: 3 in, 3 out]
            }
            frame True {
            }
          }
          n470 = local read "Abort"() -> (w1085:bool)
          n471 = property on="Bias On/Off:" class="Bool (strict)"() -> ("Blinking"=w1084:bool)  [unwired: 2 in, 2 out]
          n472 = Not Or(1:w1085, 2:w1084) -> (0:w1083:bool)
          n473 = Build Array(w1083, w1084, w1085) -> (w1086:bool[])
          n474 = Search 1D Array(1D array=w1086, element=TRUE) -> (index of element=w1088:i32)  [unwired: 1 in]
          n475 = Increment(x=w1088) -> (x+1=w1074:i32)
          n476 = Pick Line(multi-line string=" null\n Run ended normally.\n Compliance exceeded. \n Run aborted early.", line index=w1074) -> (output string=w1075:string)  [unwired: 1 in]
          n477 = global read "QC_RunInformation.vi" "Run info"() -> (w1077:T10)
          n478 = Bundle By Name(cluster=w1077, "End of Run comment:"=w1075) -> (w1076:T10)
          n479 = global write "QC_RunInformation.vi" "Run info"(w1076) -> ()
          n480 = Concatenate Strings(" End of Run.", "\r\n", w1075) -> (w1078:string)
          n481 = Concatenate Strings(w1075, "\r\n", "RAMPING DOWN VOLTS") -> (w1081:string)
          n482 = stacked-sequence {
            tunnel: w1081 -> [w1101 _ _ _]
            tunnel: w1078 -> [_ _ w1105 _]
            frame #0 {
              n483 = local write "Status:"(w1101) -> ()
            }
            frame #1 {
              n484 = local read "Simulation?"() -> (w1102:bool)
              n485 = case shown="False" w1102 {
                frame False {
                  n486 = global read "QC_MeasurementSetup.vi" "Striptest Measurement Parameters"() -> (w1104:T8)
                  n487 = Unbundle By Name(w1104) -> ("SMU"=w1103:refnum<class "SupplyControl.lvclass">)
                  n488 = call-dynamic "Supply_Stby.vi"("SupplyControl in"=w1103) -> ()  [unwired: 9 in, 2 out]
                }
                frame True {
                }
              }
            }
            frame #2 {
              n489 = local write "Status:"(w1105) -> ()
            }
            frame #3 {
              w1108 = 0
              n490 = property on="Save Data" class="Bool (strict)"("DisabledEnum"=w1108) -> ()  [unwired: 2 in, 2 out]
              n491 = property on="Quit w/o saving" class="Bool (strict)"("DisabledEnum"=w1108) -> ()  [unwired: 2 in, 2 out]
              n492 = property on="ReCheck" class="Bool"("DisabledEnum"=w1108) -> ()  [unwired: 2 in, 2 out]
              n493 = property on="Auto ReCheck" class="Bool (strict)"("DisabledEnum"=1) -> ()  [unwired: 2 in, 2 out]
              n494 = local write "Status:"("Run finished. \nSave data?" ("STATUS 1")) -> ()
            }
          }
        }
        frame #6 {
          w1120 = ""
          n495 = stacked-sequence {
            tunnel: [w1142 _ _ _] -> w1138
            tunnel: [w1141 _ _ _] -> w1137
            tunnel: w1131 -> [_ w1245 w1260 _]
            tunnel: w1130 -> [w1140 _ _ _]
            frame #0 {
              # "Loop and await decision on whether to save or junk data"
              n496 = local read "Show:"() -> (w1143:u16)
              n497 = while {
                shift-right: [w1151] -> _
                shift-left: w1143 -> [w1152]
                tunnel: ["Save Data"] -> w1141
                tunnel: ["Quit w/o saving"] -> w1142
                tunnel: w1140 -> [w1144]
                stop <- w1155 stop-if-true
                # "display data if selected region changes"
                n498 = Wait (ms)(milliseconds to wait=u32 200) -> ()  [unwired: 1 out]
                n499 = local read "Show:"() -> (w1153:u16)
                n500 = Not Equal?(x=w1153, y=w1152) -> (x != y?=w1154:bool)
                n501 = Or(x="ReCheck", y="Auto ReCheck") -> (x .or. y?=w1146:bool)
                n502 = case shown="True" w1146 {
                  tunnel: "Auto ReCheck" -> [_ w1157]
                  tunnel: w1144 -> [_ w1156]
                  frame False {
                  }
                  frame True {
                    n503 = case shown="True" w1157 {
                      tunnel: w1156 -> [_ w1187]
                      frame False {
                        n504 = local read "probe points per region"() -> (w1164:i32[])
                        n505 = local read "Region Indices"() -> (w1165:i32[])
                        n506 = local read "Show:"() -> (w1163:u16)
                        n507 = Index Array(array=w1165, index=w1163) -> (element=w1162:i32)
                        n508 = Index Array(array=w1164, index=w1163) -> (element=w1161:i32)
                        n509 = flat-sequence {
                          tunnel: w1162 -> [w1166]
                          tunnel: w1161 -> [w1170]
                          tunnel: [w1166] -> w1160
                          tunnel: [w1170] -> w1159
                          tunnel: [w1169] -> w1158
                          tunnel: w1160 -> [w1186]
                          tunnel: w1159 -> [w1183]
                          tunnel: w1158 -> [w1172]
                          frame #0 {
                            n510 = local read "Probe Card Channels"() -> (w1167:i32)
                            n511 = local read "Auto ReCheck"() -> (w1168:bool)
                            n512 = local read "Thresholds:"() -> (w1171:T2)
                            n513 = call "ReCheckStrips.vi"("Probe Card Channels"=w1167, "Auto Re-Check"=w1168, "Thresholds"=w1171, "region in"=w1166, "Number of strips probed"=w1170) -> ("Thresholds copy"=w1169:T17)  [unwired: 6 in]
                            n514 = local write "Thresholds:"(w1169) -> ()
                          }
                          frame #1 {
                            n515 = local read "max scale array"() -> (w1185:i32[])
                            n516 = local read "min scale array"() -> (w1184:i32[])
                            n517 = call "DisplayStriptestData.vi"("min scale array"=w1184, "max scale array"=w1185, "# probed"=w1183, "Display Stats?"=TRUE, "Thresholds"=w1172, "Region"=w1186) -> ("Defects"=w1178:i32[][], "Resistance [MW]"=w1179:cluster{u32, i32, "Array OUT":dbl[]}, "Capacitance [pF]"=w1181:cluster{u32, i32, "Array OUT":dbl[]}, "Current [nA]"=w1180:cluster{u32, i32, "Array OUT":dbl[]}, "Strip Quality Data"=w1177:T16)
                            n518 = Unbundle By Name(w1177) -> ("pass Rate in %"=w1176:dbl, "Bad channel list"=w1175:i32[], "No of bad strips"=w1174:i32, "Defect description list"=w1173:i32[])
                            n519 = local write "Current [nA]"(w1180) -> ()
                            n520 = local write "Capacitance [pF]"(w1181) -> ()
                            n521 = local write "Resistance [MW]"(w1179) -> ()
                            n522 = local write "Defects"(w1178) -> ()
                            n523 = local write "% OK:"(w1176) -> ()
                            n524 = local write "Bad Strip List"(w1175) -> ()
                            n525 = local write "# total defects:"(w1174) -> ()
                            n526 = local write "defect type array"(w1173) -> ()
                          }
                        }
                      }
                      frame True {
                        n527 = flat-sequence {
                          tunnel: w1187 -> [w1188]
                          frame #0 {
                            n528 = local read "Region Indices"() -> (w1189:i32[])
                            n529 = Array Size(array=w1189) -> (size(s)=w1190:i32)
                            n530 = for {
                              N: w1190 -> [_]
                              tunnel: w1189 -> [w1192] mode=indexing
                              tunnel: w1188 -> [w1191] mode=indexing
                              n531 = case shown="True" w1191 {
                                tunnel: w1192 -> [_ w1196]
                                frame False {
                                }
                                frame True {
                                n532 = local read "probe points per region"() -> (w1198:i32[])
                                n533 = Index Array(array=w1198, index=w1196) -> (element=w1197:i32)
                                n534 = flat-sequence {
                                tunnel: w1196 -> [w1203]
                                tunnel: w1197 -> [w1202]
                                tunnel: [w1203] -> w1195
                                tunnel: [w1202] -> w1194
                                tunnel: [w1201] -> w1193
                                tunnel: w1195 -> [w1219]
                                tunnel: w1194 -> [w1216]
                                tunnel: w1193 -> [w1205]
                                frame #0 {
                                n535 = local read "Probe Card Channels"() -> (w1199:i32)
                                n536 = local read "Auto ReCheck"() -> (w1200:bool)
                                n537 = local read "Thresholds:"() -> (w1204:T2)
                                n538 = call "ReCheckStrips.vi"("Probe Card Channels"=w1199, "Auto Re-Check"=w1200, "Thresholds"=w1204, "region in"=w1203, "Number of strips probed"=w1202) -> ("Thresholds copy"=w1201:T17)  [unwired: 6 in]
                                n539 = local write "Thresholds:"(w1201) -> ()
                                }
                                frame #1 {
                                n540 = local read "max scale array"() -> (w1218:i32[])
                                n541 = local read "min scale array"() -> (w1217:i32[])
                                n542 = call "DisplayStriptestData.vi"("min scale array"=w1217, "max scale array"=w1218, "# probed"=w1216, "Display Stats?"=TRUE, "Thresholds"=w1205, "Region"=w1219) -> ("Defects"=w1211:i32[][], "Resistance [MW]"=w1212:cluster{u32, i32, "Array OUT":dbl[]}, "Capacitance [pF]"=w1214:cluster{u32, i32, "Array OUT":dbl[]}, "Current [nA]"=w1213:cluster{u32, i32, "Array OUT":dbl[]}, "Strip Quality Data"=w1210:T16)
                                n543 = Unbundle By Name(w1210) -> ("pass Rate in %"=w1209:dbl, "Bad channel list"=w1208:i32[], "No of bad strips"=w1207:i32, "Number of defects per category"=w1206:i32[])
                                n544 = local write "Current [nA]"(w1213) -> ()
                                n545 = local write "Capacitance [pF]"(w1214) -> ()
                                n546 = local write "Resistance [MW]"(w1212) -> ()
                                n547 = local write "Defects"(w1211) -> ()
                                n548 = local write "% OK:"(w1209) -> ()
                                n549 = local write "Bad Strip List"(w1208) -> ()
                                n550 = local write "# total defects:"(w1207) -> ()
                                n551 = local write "defect type array"(w1206) -> ()
                                }
                                }
                                }
                              }
                            }
                          }
                          frame #1 {
                            n552 = local write "Auto ReCheck"(FALSE) -> ()
                          }
                        }
                      }
                    }
                  }
                }
                n553 = case shown="True" w1154 {
                  tunnel: w1153 -> [w1221 w1228]
                  tunnel: [w1221 w1228] -> w1151
                  frame False {
                  }
                  frame True {
                    n554 = local read "probe points per region"() -> (w1238:i32[])
                    n555 = local read "Region Indices"() -> (w1229:i32[])
                    n556 = local read "max scale array"() -> (w1239:i32[])
                    n557 = local read "min scale array"() -> (w1240:i32[])
                    n558 = local read "Thresholds:"() -> (w1243:T2)
                    n559 = Index Array(array=w1229, index=w1228) -> (element=w1227:i32)
                    n560 = Index Array(array=w1238, index=w1228) -> (element=w1244:i32)
                    n561 = Index Array(array=w1239, index=w1228) -> (element=w1226:i32)
                    n562 = Index Array(array=w1240, index=w1228) -> (element=w1225:i32)
                    n563 = call "DisplayStriptestData.vi"("min scale array"=w1240, "max scale array"=w1239, "# probed"=w1244, "Display Stats?"=TRUE, "Thresholds"=w1243, "Region"=w1227) -> ("Defects"=w1241:i32[][], "Resistance [MW]"=w1235:cluster{u32, i32, "Array OUT":dbl[]}, "Capacitance [pF]"=w1236:cluster{u32, i32, "Array OUT":dbl[]}, "Current [nA]"=w1237:cluster{u32, i32, "Array OUT":dbl[]}, "Strip Quality Data"=w1242:T16)
                    n564 = Increment(x=w1226) -> (x+1=w1223:i32)
                    n565 = Increment(x=w1225) -> (x+1=w1224:i32)
                    n566 = property on="Resistance [MW]" class="WFGraph (strict)"("XScale.Minimum"=w1224) -> ()  [unwired: 2 in, 2 out]
                    n567 = property on="Resistance [MW]" class="WFGraph (strict)"("XScale.Maximum"=w1223) -> ()  [unwired: 2 in, 2 out]
                    n568 = property on="Current [nA]" class="WFGraph (strict)"("XScale.Maximum"=w1223) -> ()  [unwired: 2 in, 2 out]
                    n569 = Unbundle By Name(w1242) -> ("pass Rate in %"=w1232:dbl, "Bad channel list"=w1230:i32[], "No of bad strips"=w1233:i32, "Number of defects per category"=w1231:i32[])
                    n570 = property on="Capacitance [pF]" class="WFGraph (strict)"("XScale.Minimum"=w1224) -> ()  [unwired: 2 in, 2 out]
                    n571 = property on="Defects" class="IntGraph (strict)"("XScale.Minimum"=w1224) -> ()  [unwired: 2 in, 2 out]
                    n572 = local write "Current [nA]"(w1237) -> ()
                    n573 = local write "Capacitance [pF]"(w1236) -> ()
                    n574 = property on="Current [nA]" class="WFGraph (strict)"("XScale.Minimum"=w1224) -> ()  [unwired: 2 in, 2 out]
                    n575 = local write "Resistance [MW]"(w1235) -> ()
                    n576 = local write "Defects"(w1241) -> ()
                    n577 = property on="Capacitance [pF]" class="WFGraph (strict)"("XScale.Maximum"=w1223) -> ()  [unwired: 2 in, 2 out]
                    n578 = Increment(x=w1223) -> (x+1=w1222:i32)
                    n579 = property on="Defects" class="IntGraph (strict)"("XScale.Maximum"=w1222) -> ()  [unwired: 2 in, 2 out]
                    n580 = local write "% OK:"(w1232) -> ()
                    n581 = local write "Bad Strip List"(w1230) -> ()
                    n582 = local write "# total defects:"(w1233) -> ()
                    n583 = local write "defect type array"(w1231) -> ()
                  }
                }
                n584 = Or(x="Save Data", y="Quit w/o saving") -> (x .or. y?=w1155:bool)
              }
              n585 = local write "Save Data"("Auto quit &\nswitch off bias") -> ()
            }
            frame #1 {
              n586 = case shown="False" w1245 {
                frame False {
                  # "supply to standby"
                  n587 = global read "QC_MeasurementSetup.vi" "Striptest Measurement Parameters"() -> (w1257:T8)
                  n588 = Unbundle By Name(w1257) -> ("Bias Supply"=w1246:refnum<class "SupplyControl.lvclass">, "Measurement switch"=w1256:refnum<class "Switching.lvclass">)
                  n589 = local read "Current Bias Voltage [V]"() -> (w1250:dbl)
                  n590 = call-dynamic "MatrixSwitch.vi"("Action"=T6."Reset", "Switching in"=w1256) -> ("error out"=w1255:errorcluster)  [unwired: 7 in, 2 out]
                  n591 = call "SupplyRamp.vi"("error in"=w1255, "Requested Voltage"=0.0, "Step Size"=10.0, "Step Delay"=1000, "Supply IN"=w1246, "Starting Voltage"=w1250) -> ("error out"=w1253:errorcluster, "Supply OUT"=w1252:refnum<class "SupplyControl.lvclass">, "Current Voltage"=w1251:dbl)  [unwired: 2 in, 1 out]
                  n592 = local write "Current Bias Voltage [V]"(w1251) -> ()
                  n593 = call-dynamic "Supply_Stby.vi"("error in (no error)"=w1253, "SupplyControl in"=w1252) -> ()  [unwired: 8 in, 2 out]
                }
                frame True {
                }
              }
            }
            frame #2 {
              n594 = case shown="False" w1260 {
                frame False {
                  n595 = global read "QC_MeasurementSetup.vi" "Striptest Measurement Parameters"() -> (w1262:T8)
                  n596 = Unbundle By Name(w1262) -> ("Arduino"=w1267:refnum<class "ArduinoControl.lvclass">)
                  n597 = local read "Temperature Progression"() -> (w1272:T3)
                  n598 = local read "Run Duration:"() -> (w1269:string)
                  n599 = call "ArduinoRead.vi"("Arduino function"=enum16{"T/RH", "Interlock", "Edgesense"}."T/RH", "ArduinoControl in"=w1267) -> ("error out"=w1273:errorcluster, "Temperature [°C]"=w1264:dbl, "ArduinoControl out"=w1274:refnum<class "ArduinoControl.lvclass">)  [unwired: 4 in, 3 out]
                  "Last Temperature [°C]" <- w1264
                  n600 = call "ArduinoClose.vi"("error in (no error)"=w1273, "ArduinoControl in"=w1274) -> ()  [unwired: 8 in, 2 out]
                  n601 = Unbundle(w1272) -> ("Time Array"=w1270:string[], "Temperature Array [°C]"=w1265:dbl[])  [unwired: 1 out]
                  n602 = Build Array (concatenate)(w1270, w1269) -> (w1268:string[])
                  n603 = Build Array (concatenate)(w1265, w1264) -> (w1263:dbl[])
                  n604 = Bundle(cluster=w1272, "Time Array"=w1268, "Temperature Array [°C]"=w1263) -> (w1271:T3)  [unwired: 1 in]
                  n605 = local write "Temperature Progression"(w1271) -> ()
                }
                frame True {
                }
              }
              n606 = local read "# probed"() -> (w1259:i32)
              n607 = call "SaveJPEG.vi"("Picture No."=w1259, "Test"="Striptest") -> ()  [unwired: 1 in, 2 out]
              n608 = One Button Dialog(message="Please switch bias off NOW and then open\nprobestation enclosure and raise needle.") -> ()  [unwired: 1 in, 1 out]
            }
            frame #3 {
              n609 = One Button Dialog(message="Please ensure detector bias is OFF!") -> ()  [unwired: 1 in, 1 out]
            }
          }
          n610 = case shown="True" w1138 {
            tunnel: [FALSE w1378] -> w1136
            frame False {
            }
            frame True {
              n611 = Two Button Dialog(message="Are you sure you don't want to save the data?", 1:"Quit" ("F button name (\"Cancel\")"), 2:"Save data" ("T button name (\"OK\")")) -> (T button?=w1378:bool)
            }
          }
          n612 = global read "ProbePlanParams.vi" "ProbePlan Parameters IN"() -> (w1135:T11)
          n613 = Unbundle By Name(w1135) -> ("Test ProbePoints.Regions Enabled"=w1133:bool[], "ProbePlan array"=w1132:T12)
          n614 = Or(x=w1137, y=w1136) -> (x .or. y?=w1126:bool)
          n615 = Array Size(array=w1133) -> (size(s)=w1134:i32)
          n616 = case shown="True" w1126 {
            tunnel: w1134 -> [w1282 w1310]
            tunnel: w1133 -> [w1281 w1309]
            tunnel: w1132 -> [_ w1308]
            tunnel: [w1277 w1306] -> w1129
            tunnel: [w1279 w1304] -> w1128
            tunnel: ["" w1301] -> w1127
            frame False {
              n617 = for {
                N: w1282 -> [_]
                tunnel: w1281 -> [w1286] mode=indexing
                tunnel: [w1285] -> w1280 mode=indexing
                tunnel: [w1284] -> w1278 mode=indexing
                i -> [w1283]
                n618 = case shown="True" w1286 {
                  tunnel: [100.0 w1291] -> w1285
                  tunnel: [TRUE w1290] -> w1284
                  tunnel: w1283 -> [_ w1289]
                  frame False {
                  }
                  frame True {
                    n619 = local read "probe points per region"() -> (w1297:i32[])
                    n620 = local read "max scale array"() -> (w1296:i32[])
                    n621 = local read "min scale array"() -> (w1295:i32[])
                    n622 = local read "Thresholds:"() -> (w1299:T2)
                    n623 = Index Array(array=w1297) -> (element=w1293:i32)  [unwired: 1 in]
                    n624 = call "DisplayStriptestData.vi"("min scale array"=w1295, "max scale array"=w1296, "# probed"=w1293, "Display Stats?"=TRUE, "Thresholds"=w1299, "Region"=w1289) -> ("Strip Quality Data"=w1294:T16)  [unwired: 4 out]
                    n625 = Unbundle By Name(w1294) -> ("pass Rate in %"=w1291:dbl)
                    n626 = Greater?(x=w1291, y=98.0) -> (0:w1290:bool)
                  }
                }
              }
              n627 = And Array Elements(Boolean array=w1278) -> (logical AND=w1277:bool)
              n628 = Array Max & Min(array=w1280) -> (min value=w1279:dbl)  [unwired: 3 out]
            }
            frame True {
              n629 = for {
                N: w1310 -> [_]
                tunnel: w1309 -> [w1320] mode=indexing
                tunnel: w1308 -> [w1319] mode=indexing
                tunnel: [w1311] -> w1307 mode=indexing
                tunnel: [w1317] -> w1305 mode=indexing
                tunnel: [w1316] -> w1303
                shift-right: [w1315] -> w1300
                shift-left: _ -> [w1312]
                i -> [w1318]
                n630 = case shown="False" w1320 {
                  tunnel: w1318 -> [_ w1333]
                  tunnel: w1319 -> [_ w1332]
                  tunnel: [100.0 w1329] -> w1317
                  tunnel: [w1322 w1328] -> w1316
                  tunnel: [w1322 w1327] -> w1313
                  tunnel: [TRUE w1324] -> w1311
                  frame False {
                    w1322 = ""
                  }
                  frame True {
                    n631 = Unbundle By Name(w1332) -> ("Region"=w1331:string)
                    n632 = flat-sequence {
                      tunnel: w1333 -> [w1335]
                      tunnel: w1331 -> [w1337]
                      tunnel: [w1335] -> w1330
                      tunnel: [w1339] -> w1328
                      tunnel: [w1338] -> w1327
                      tunnel: [w1337] -> w1326
                      tunnel: [w1334] -> w1325
                      tunnel: w1330 -> [w1364]
                      tunnel: [w1369] -> w1329
                      tunnel: w1326 -> [_]
                      tunnel: w1325 -> [w1368]
                      tunnel: [w1363] -> w1324
                      frame #0 {
                        (unwired) "ProbeplanIndex Current PinholeFlag Capacitance Resistance" ("Array Titles")
                        w1353 = T5."Read Array" ("Action")
                        n633 = Concatenate Strings("Saving data for " ("string"), w1337) -> (w1362:string)
                        n634 = local write "Status:"(w1362) -> ()
                        n635 = call "MultiRegionData.vi"("Action"=w1353, "Array No."=4, "Region index"=w1335) -> ("Array OUT"=w1351:dbl[])  [unwired: 3 in, 1 out]
                        n636 = local read "Temperature Progression"() -> (w1342:T3)
                        n637 = Multiply(x=w1351, y=0.001) -> (x*y=w1350:dbl[])
                        n638 = call "MultiRegionData.vi"("Action"=w1353, "Array No."=0, "Region index"=w1335) -> ("Array OUT"=w1346:dbl[])  [unwired: 3 in, 1 out]
                        n639 = call "MultiRegionData.vi"("Action"=w1353, "Array No."=1, "Region index"=w1335) -> ("Array OUT"=w1347:dbl[])  [unwired: 3 in, 1 out]
                        n640 = call "MultiRegionData.vi"("Action"=w1353, "Array No."=3, "Region index"=w1335) -> ("Array OUT"=w1349:dbl[])  [unwired: 3 in, 1 out]
                        n641 = call "MultiRegionData.vi"("Array No."=2, "Region index"=w1335) -> ("Array OUT"=w1348:dbl[])  [unwired: 4 in, 1 out]
                        n642 = Unbundle By Name(w1342) -> ("Temperature Array [°C]"=w1341:dbl[], "Humidity Array [RH %]"=w1340:dbl[])
                        n643 = Build Array(w1346, w1347, w1348, w1349, w1350) -> (w1345:dbl[][])
                        n644 = call <vilib>:"Std Deviation and Variance.vi"("X"=w1341) -> ("mean"=w1344:dbl)  [unwired: 1 in, 2 out]
                        n645 = call <vilib>:"Std Deviation and Variance.vi"("X"=w1340) -> ("mean"=w1343:dbl)  [unwired: 1 in, 2 out]
                        n646 = Transpose 2D Array(2D array=w1345) -> ()  [unwired: 1 out]
                        n647 = call "SaveDataFile.vi"("Temperature"=w1344, "Run uninterrupted?"=FALSE, "Humidity"=w1343, "Sensor Index/\nSegment No."=w1335, "Array Titles"="ProbeplanIndex Current Capacitance Resistance", "Strip Segment"=w1337, "Arrays format"="%016.6f") -> ("Filename OUT"=w1338:string, "Pathname OUT"=w1339:string, "Path + Filename OUT"=w1334:string)  [unwired: 5 in, 1 out]
                      }
                      frame #1 {
                        n648 = local read "probe points per region"() -> (w1374:i32[])
                        n649 = local read "max scale array"() -> (w1373:i32[])
                        n650 = local read "min scale array"() -> (w1372:i32[])
                        n651 = local read "Thresholds:"() -> (w1376:T2)
                        n652 = Index Array(array=w1374, index=w1364) -> (element=w1370:i32)
                        n653 = call "DisplayStriptestData.vi"("min scale array"=w1372, "max scale array"=w1373, "# probed"=w1370, "Display Stats?"=TRUE, "Thresholds"=w1376, "Region"=w1364) -> ("Strip Quality Data"=w1371:T16)  [unwired: 4 out]
                        n654 = Unbundle By Name(w1371) -> ("pass Rate in %"=w1369:dbl, "No of bad strips"=w1367:i32, "Bad channel list"=w1366:i32[], "Defect description list"=w1365:i32[])
                        n655 = call "CreateDefectFile.vi"("Region"=w1364, "Pass rate"=w1369, "Defect description list"=w1365, "Bad channel array"=w1366, "No of bad strips"=w1367, "Filename IN"=w1368) -> ("passed"=w1363:bool)  [unwired: 4 in, 1 out]
                      }
                    }
                  }
                }
                n656 = call <vilib>:"Space Constant.vi"() -> ("String"=w1314:string)
                n657 = Concatenate Strings(w1312, w1314, w1313) -> (w1315:string)
              }
              n658 = Array Max & Min(array=w1305) -> (min value=w1304:dbl)  [unwired: 3 out]
              n659 = And Array Elements(Boolean array=w1307) -> (logical AND=w1306:bool)
              "Module failed/passed" <- w1306
              n660 = call <vilib>:"Space Constant.vi"() -> ("String"=w1302:string)
              n661 = Concatenate Strings(w1303, w1302, w1300) -> (w1301:string)
            }
          }
          n662 = local read "Temperature Progression"() -> (w1125:T3)
          n663 = Unbundle By Name(w1125) -> ("Temperature Array [°C]"=w1123:dbl[], "Humidity Array [RH %]"=w1124:dbl[])
          n664 = call <vilib>:"Std Deviation and Variance.vi"("X"=w1123) -> ("standard deviation"=w1117:dbl)  [unwired: 1 in, 2 out]
          n665 = call <vilib>:"Std Deviation and Variance.vi"("X"=w1124) -> ("standard deviation"=w1116:dbl)  [unwired: 1 in, 2 out]
          n666 = Greater?(x=w1117, y=5) -> (0:w1114:bool)
          n667 = Greater?(x=w1116, y=10) -> (0:w1115:bool)
          n668 = Select(t="large temperature fluctuations", s=w1114, f=w1120) -> (s? t:f=w1111:string)
          n669 = Select(t="large humidity fluctuations", s=w1115, f=w1120) -> (s? t:f=w1112:string)
          n670 = Concatenate Strings(w1111, "\t", w1112) -> (w1110:string)
          n671 = call "WriteLogFile.vi"("Run uninterrupted?"=FALSE, "Automatic warning"=w1110, "Data File"=w1127, "DUT passed?"=w1129, "Value TechSpec criteria"=w1128, "Files saved?"=w1126) -> ()  [unwired: 5 in, 1 out]
        }
      }
    }
  }
